vi "模拟发送.vi"() -> ()   [LabVIEW 2013]
panel:
  in  "循环发送帧间隔":dbl
  out "Stop":bool
  in  "内部CAN发送通道":u16(ring) items=["CAN0", "CAN1"]
  in  "加载配置文件":bool
  in  "默认":bool
  in  "开始":bool
  in  "停止":bool
  in  "选项卡控件":enum32{"从板信息", "高压板信息", "故障信息", "自定义信息发送"}(tab)
  in  "温度个数":dbl
  in  "温度":dbl
  in  "电压个数":dbl
  in  "单体电压":dbl
  in  "LIFE":i32
  in  "从板总电压":dbl
  in  "最大电压":dbl
  in  "位置":i32
  in  "最小电压":dbl
  in  "位置":i32
  in  "最大温度":dbl
  in  "位置":i32
  in  "最小温度":dbl
  in  "位置":i32
  in  "从板个数":T1(ring)
  in  "发送单体电压递增1mv":bool
  in  "发送温度递增1度":bool
  in  "板号               单体电压          电压个数":dbl[][](array[numeric])
  in  "板号          温度              温度个数":dbl[][](array[numeric])
  in  "总电压 2":dbl caption="总电压"
  in  "总电流 2":dbl caption="总电流"
  in  "外总压 2":dbl caption="外总压"
  in  "平均电流 2":dbl caption="平均电流"
  in  "充电总安时":dbl
  in  "放电总安时":dbl
  in  "发送?":bool
  in  "电压检测模块故障":enum16{"无", "一级", "二级", "三级"}(ring)
  in  "温度检测模块故障":enum16{"无", "一级", "二级", "三级"}(ring) caption="电压检测模块故障"
  in  "电流检测模块故障":enum16{"无", "一级", "二级", "三级"}(ring) caption="电压检测模块故障"
  in  "绝缘检测模块故障":enum16{"无", "一级", "二级", "三级"}(ring) caption="电压检测模块故障"
  in  "内总压检测模块故障":enum16{"无", "一级", "二级", "三级"}(ring) caption="电压检测模块故障"
  in  "外总压检测模块故障":enum16{"无", "一级", "二级", "三级"}(ring) caption="电压检测模块故障"
  in  "系统外扩时钟模块故障":enum16{"无", "一级", "二级", "三级"}(ring) caption="电压检测模块故障"
  in  "CPU内部EE故障":enum16{"无", "一级", "二级", "三级"}(ring) caption="电压检测模块故障"
  in  "EE存储器故障":enum16{"无", "一级", "二级", "三级"}(ring) caption="电压检测模块故障"
  in  "45db041存储器故障":enum16{"无", "一级", "二级", "三级"}(ring) caption="电压检测模块故障"
  in  "CPU内部FLASH存储器故障":enum16{"无", "一级", "二级", "三级"}(ring) caption="电压检测模块故障"
  in  "CPU故障":enum16{"无", "一级", "二级", "三级"}(ring) caption="电压检测模块故障"
  in  "CAN4通讯模块故障":enum16{"无", "一级", "二级", "三级"}(ring) caption="电压检测模块故障"
  in  "CAN0通讯模块故障":enum16{"无", "一级", "二级", "三级"}(ring) caption="电压检测模块故障"
  in  "CAN1通讯模块故障":enum16{"无", "一级", "二级", "三级"}(ring) caption="电压检测模块故障"
  in  "充电均衡模块故障":enum16{"无", "一级", "二级", "三级"}(ring) caption="电压检测模块故障"
  in  "放电均衡模块故障":enum16{"无", "一级", "二级", "三级"}(ring) caption="电压检测模块故障"
  in  "软件故障":enum16{"无", "一级", "二级", "三级"}(ring) caption="电压检测模块故障"
  in  "DI模块故障":enum16{"无", "一级", "二级", "三级"}(ring) caption="电压检测模块故障"
  in  "DO模块故障":enum16{"无", "一级", "二级", "三级"}(ring) caption="电压检测模块故障"
  in  "全选":bool
  in  "清空":bool
  out "硬件故障":string
  in  "循环发送":bool
  in  "单次发送":bool
  in  "自定信息CAN发送通道":u16(ring) items=["CAN0", "CAN1"]
  in  "自定义数据":string[][](table)
  in  "自定义信息CAN波特率":enum16{"250Kbps", "500Kbps"}(ring)=enum."500Kbps"
  in  "2":bool
  in  "3":bool
  in  "4":bool
  in  "5":bool
  in  "6":bool
  in  "7":bool
  in  "8":bool
  in  "9":bool
  in  "10":bool
  in  "1":bool=TRUE
  out "发送成功":bool
  in  "平均电流":dbl
  in  "外总压":dbl
  in  "总电流":dbl
  # "模拟数据发送"
  # "设置全部从板温度信息"
  # "设置全部从板电压信息"
  # "发送"
  # "双击序号可发送指定帧"
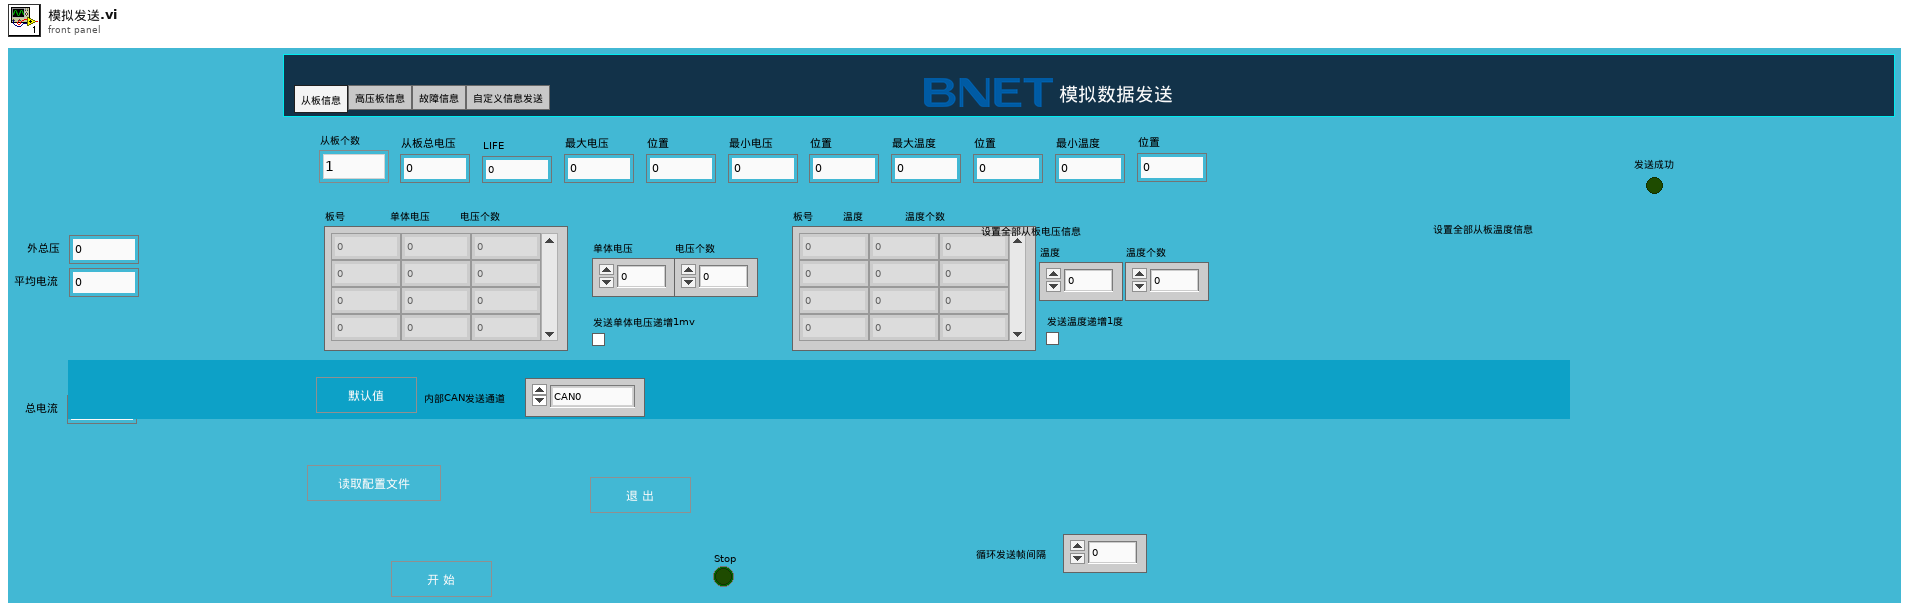
[diagram p1: front panel]
types:
  T1 = enum16{"1", "2", "3", "4", "5", "6", "7", "8", "9", "10", "11", "12", "13", "14", "15", "16", "17", "18", "19", "20", "21", "22", "23", "24", "25", "26", "27", "28", "29", "30"}
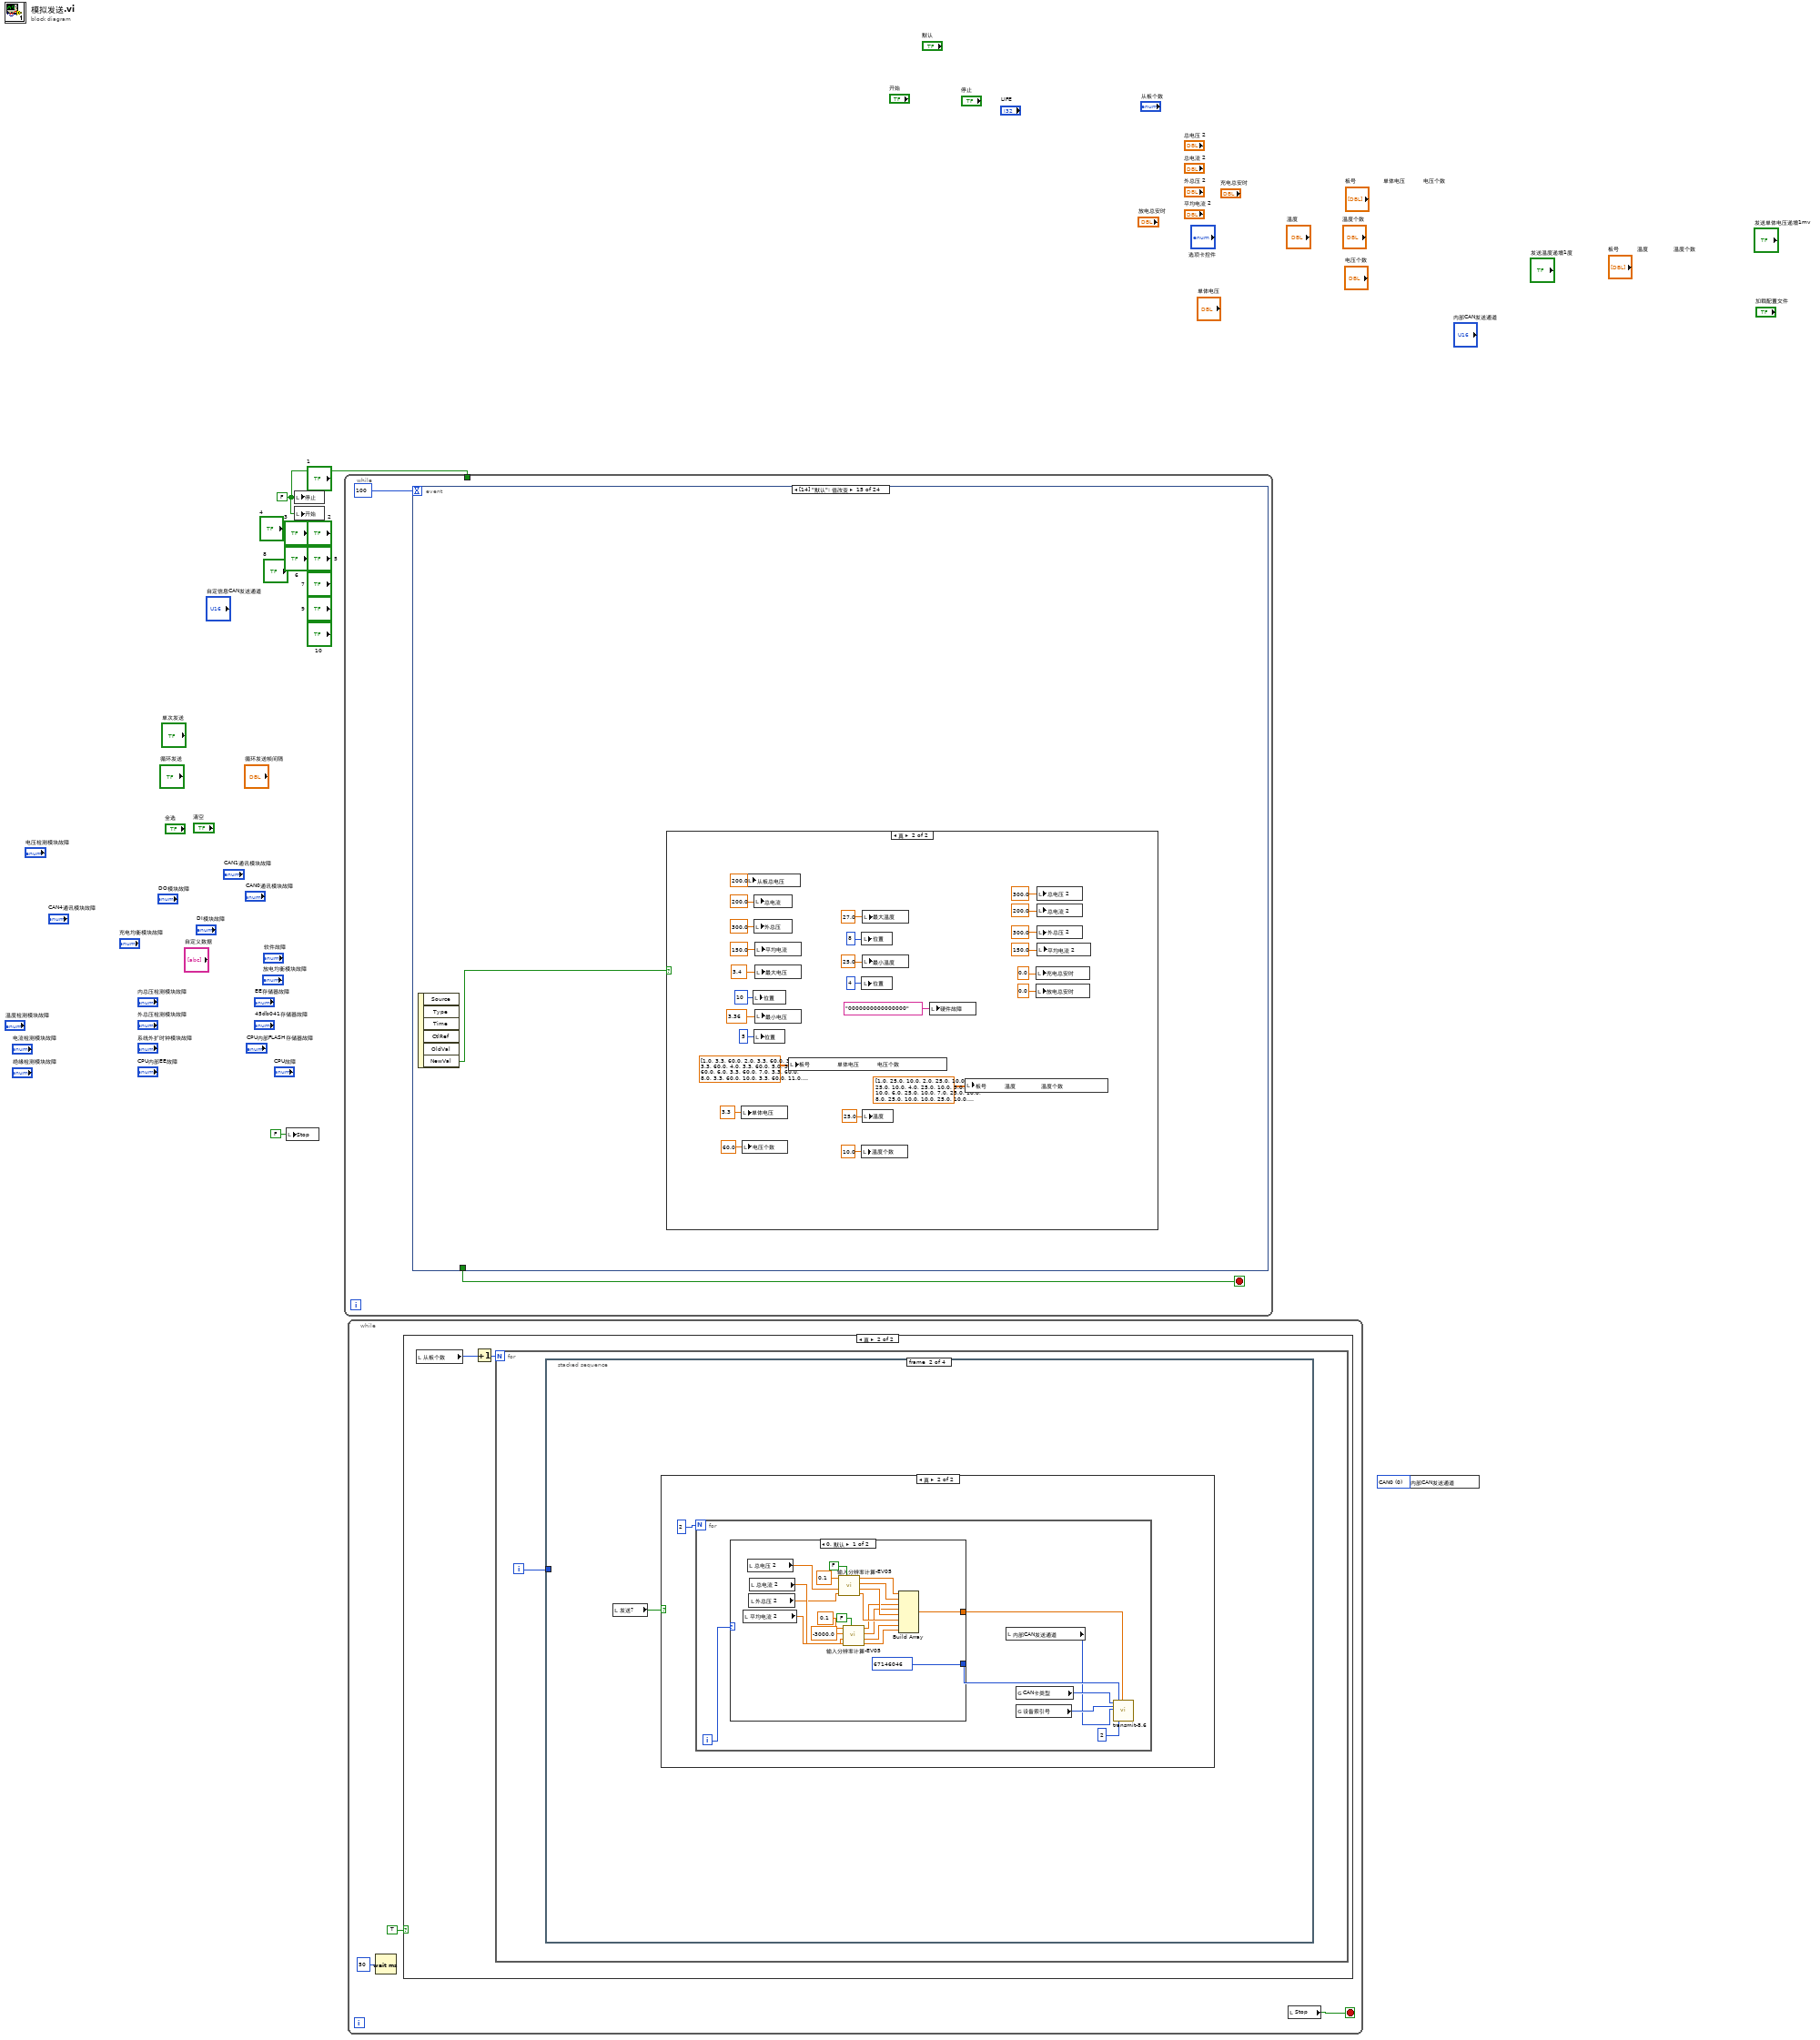
[diagram p0: block diagram]
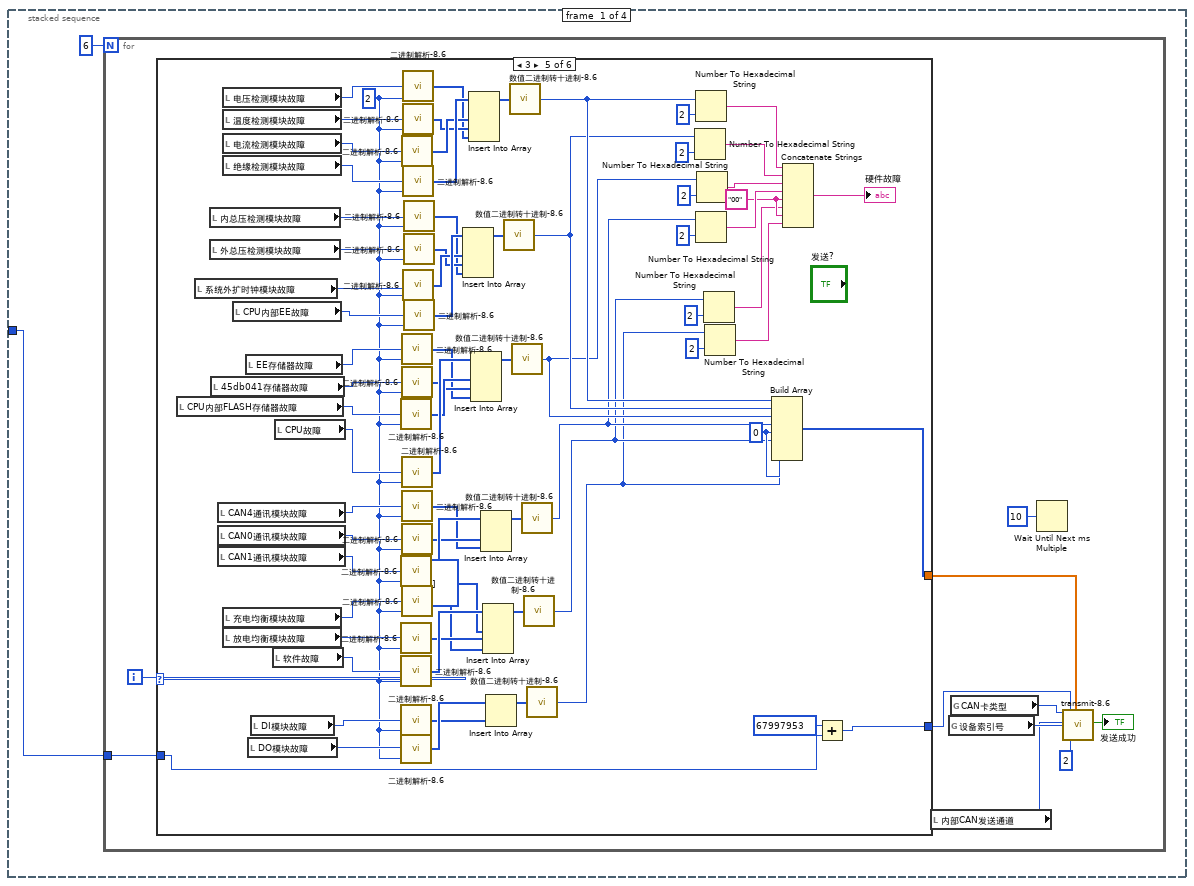
[diagram p3: hidden frame]
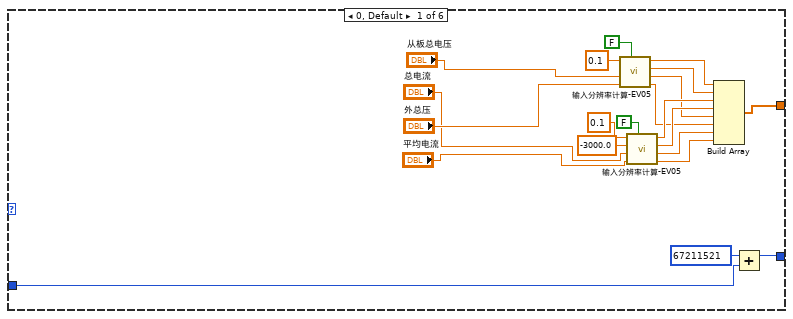
[diagram p4: hidden frame]
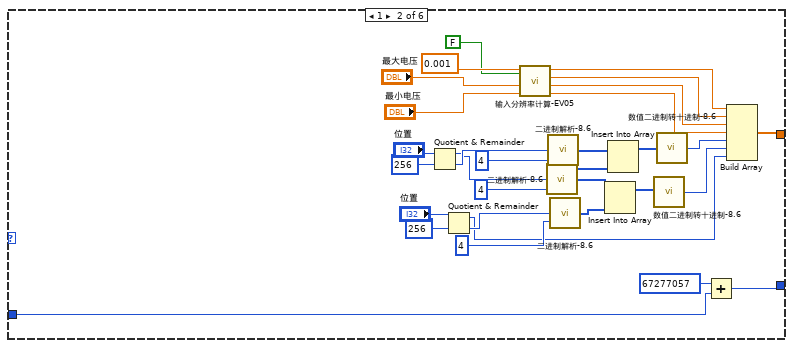
[diagram p5: hidden frame]
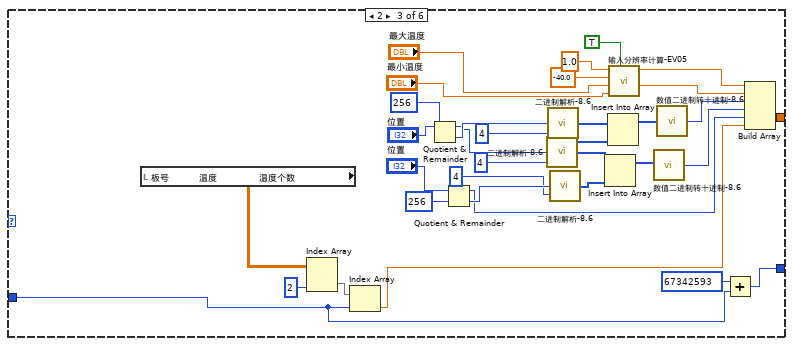
[diagram p6: hidden frame]
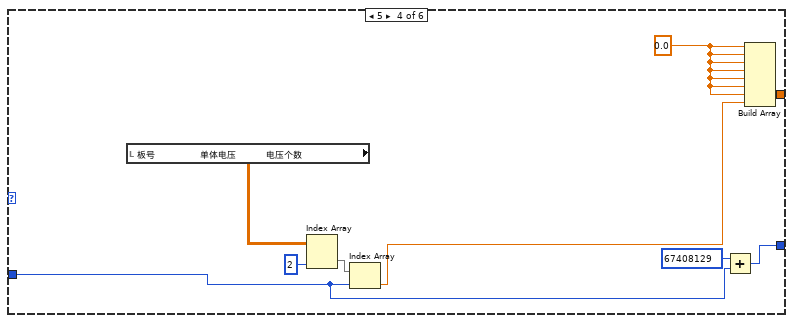
[diagram p7: hidden frame]
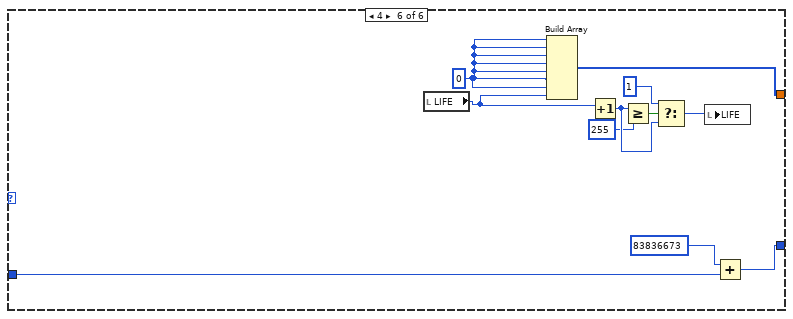
[diagram p8: hidden frame]
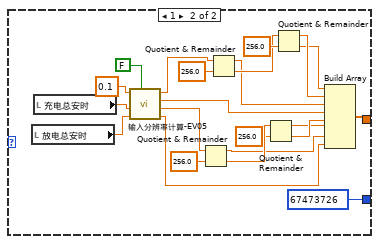
[diagram p10: hidden frame]
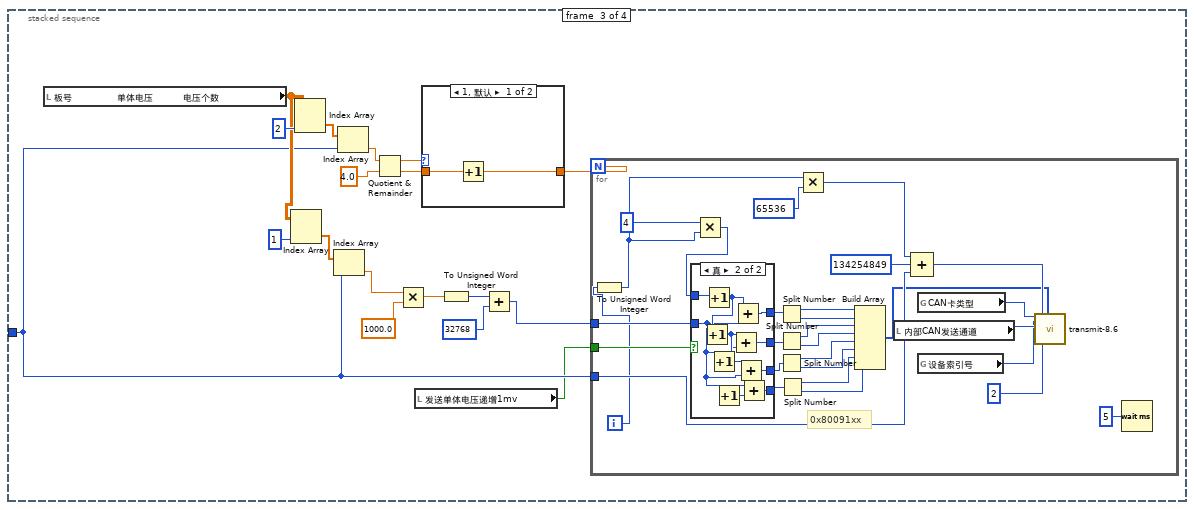
[diagram p11: hidden frame]
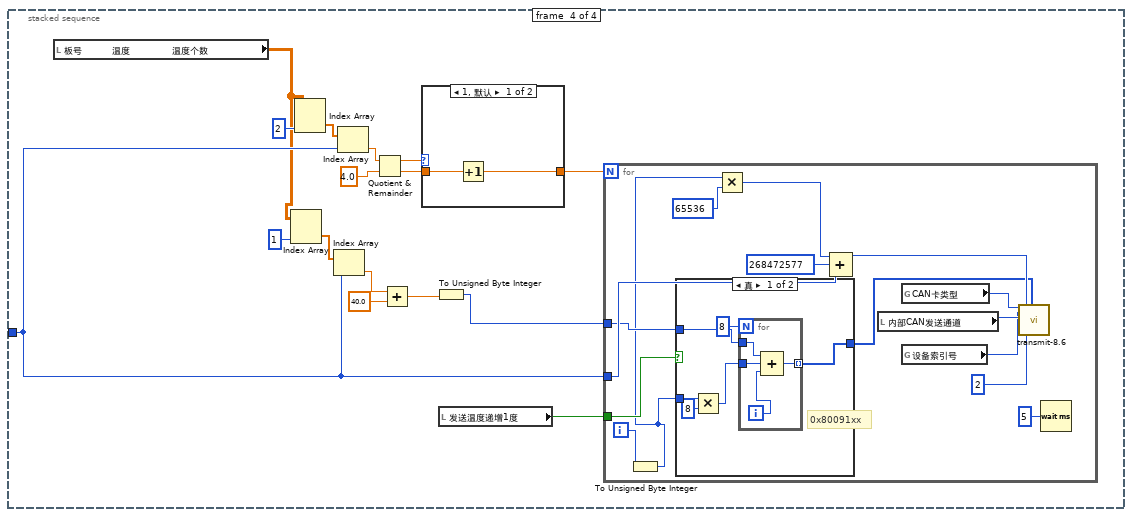
[diagram p14: hidden frame]
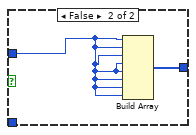
[diagram p16: hidden frame]
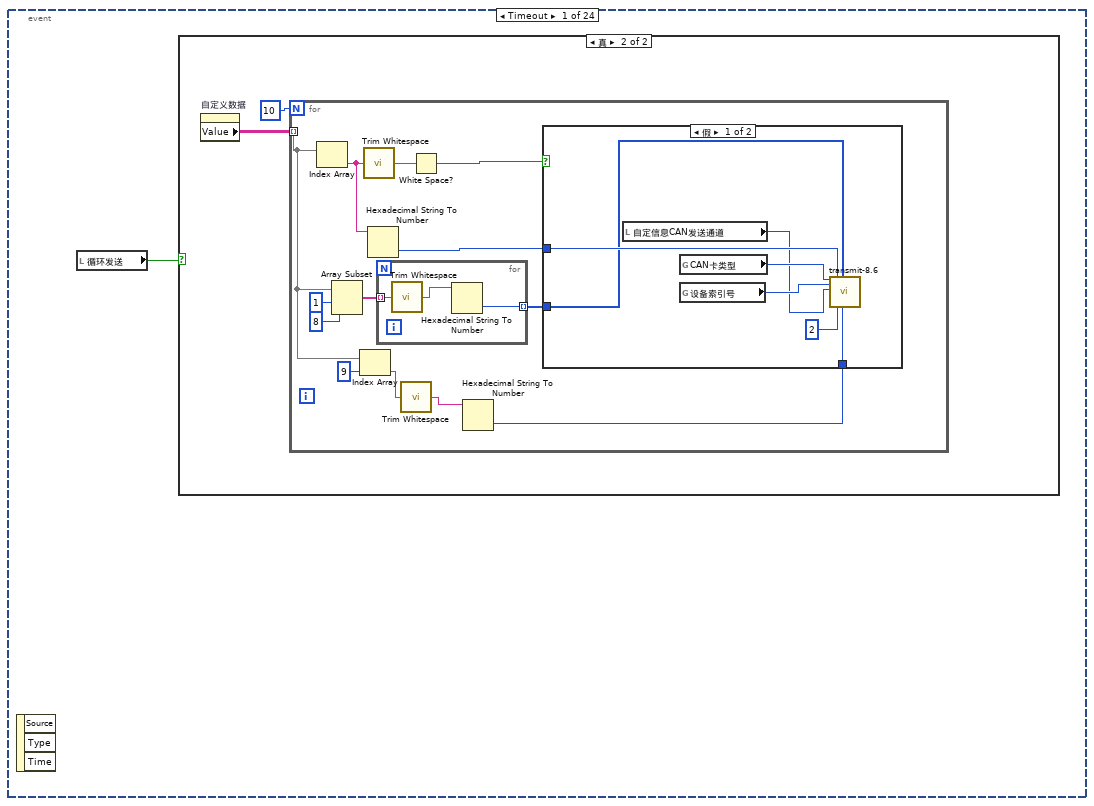
[diagram p17: hidden frame]
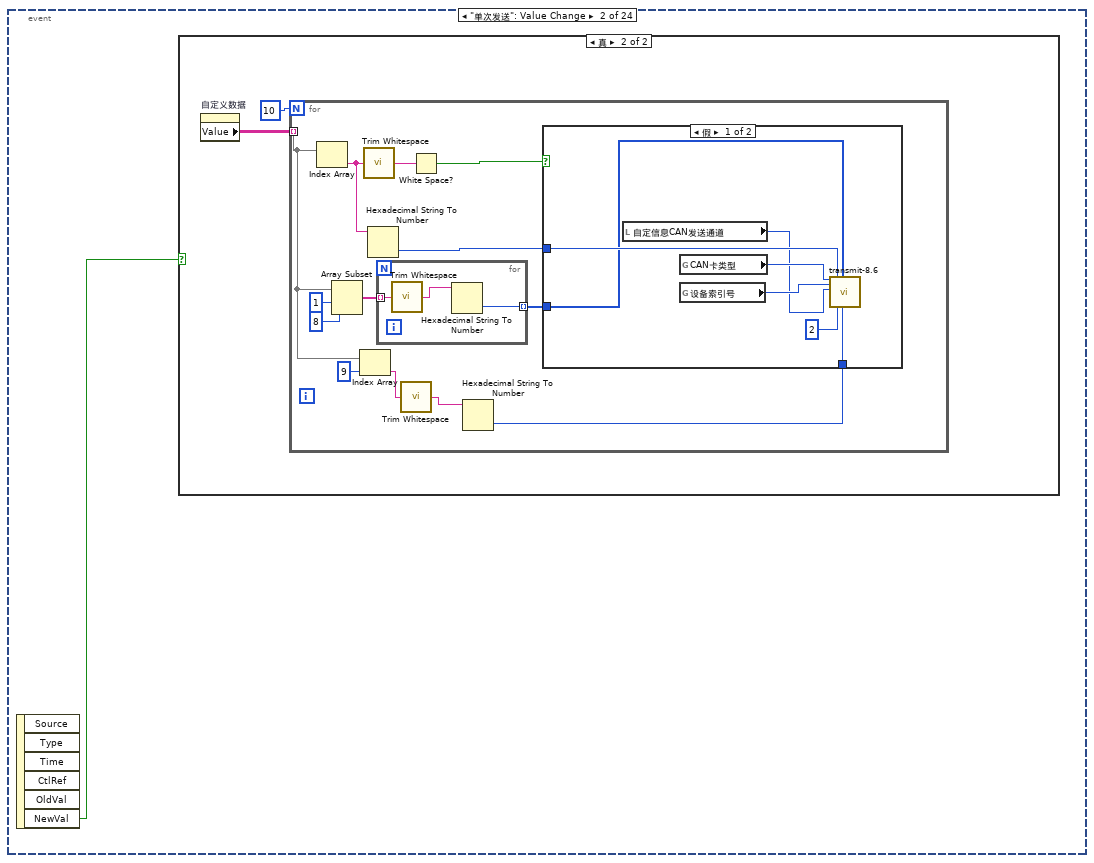
[diagram p20: hidden frame]
diagram:
  w1 = u16 0 items=["CAN0", "CAN1"] ("CAN通道")
  w3 = FALSE ("开始")
  n1 = local write "Stop"(FALSE ("Stop")) -> ()
  n2 = local write "停止"(w3) -> ()
  n3 = local write "开始"(w3) -> ()
  n4 = while {
    tunnel: w3 -> [_]
    stop <- w4 stop-if-true
    n5 = event shown="[14] \"默认\": 值改变" {
      selector: _ -> [_ _ _ _ _ _ _ _ _ _ _ _ _ _ _ _ _ _ _ _ _ _ _ _]
      dyn-events: _ -> [_ _ _ _ _ _ _ _ _ _ _ _ _ _ _ _ _ _ _ _ _ _ _ _]
      timeout: 100 -> [_ _ _ _ _ _ _ _ _ _ _ _ _ _ _ _ _ _ _ _ _ _ _ _]
      tunnel: [_ _ _ _ _ _ _ _ _ _ _ _ _ _ _ _ _ _ _ w396 TRUE ("NewVal") _ _ _] -> w4
      event Timeout {
        n6 = event-data() -> ()  [unwired: 1 in, 3 out]
        n7 = local read "循环发送"() -> (w6:bool)
        n8 = case shown="真" w6 {
          frame False {
          }
          frame True {
            n9 = property on="自定义数据" class="Tbl (严格)"() -> ("Value"=w8:string[][])  [unwired: 2 in, 2 out]
            n10 = for {
              N: 10 -> [_]
              tunnel: w8 -> [w15] mode=indexing
              n11 = Index Array(array=w15) -> (element=w18:string)  [unwired: 1 in]
              n12 = Array Subset(array=w15, index=1 ("索引"), length=8 ("长度")) -> (w10:string[])
              n13 = Index Array(array=w15, index=9 ("索引")) -> (element=w13:string)
              n14 = call <vilib>:"Trim Whitespace.vi"("string"=w18) -> ("trimmed string"=w21:string)  [unwired: 1 in]
              n15 = Hexadecimal String To Number(string=w18) -> (number=w19:u32)  [unwired: 2 in, 1 out]
              n16 = for {
                tunnel: w10 -> [w24] mode=indexing
                tunnel: [w22] -> w9 mode=indexing
                n17 = call <vilib>:"Trim Whitespace.vi"("string"=w24) -> ("trimmed string"=w23:string)  [unwired: 1 in]
                n18 = Hexadecimal String To Number(string=w23) -> (number=w22:u32)  [unwired: 2 in, 1 out]
              }
              n19 = call <vilib>:"Trim Whitespace.vi"("string"=w13) -> ("trimmed string"=w12:string)  [unwired: 1 in]
              n20 = White Space?(1:w21) -> (0:w20:bool)
              n21 = Hexadecimal String To Number(string=w12) -> (number=w11:u32)  [unwired: 2 in, 1 out]
              n22 = case shown="假" w20 {
                tunnel: w19 -> [w28 _]
                tunnel: w11 -> [w27 _]
                tunnel: w9 -> [w26 _]
                frame False {
                  n23 = local read "自定信息CAN发送通道"() -> (w25:u16)
                  n24 = global read "EV05全局变量1.vi" "CAN卡类型"() -> (w31:u32)
                  n25 = global read "EV05全局变量1.vi" "设备索引号"() -> (w30:u16)
                  n26 = call "transmit-8.6.vi"("can卡类型"=w31, "设备索引号"=w30, "CAN端口"=w25, "ID"=w28, "SendType"=u8 2, "Data"=w26, "Eflag"=w27) -> ()  [unwired: 2 in, 11 out]
                }
                frame True {
                }
              }
            }
          }
        }
      }
      event "单次发送": Value Change {
        n27 = event-data() -> ("NewVal"=w32:bool)  [unwired: 1 in, 5 out]
        n28 = case shown="真" w32 {
          frame False {
          }
          frame True {
            n29 = property on="自定义数据" class="Tbl (严格)"() -> ("Value"=w34:string[][])  [unwired: 2 in, 2 out]
            n30 = for {
              N: 10 -> [_]
              tunnel: w34 -> [w41] mode=indexing
              n31 = Index Array(array=w41) -> (element=w44:string)  [unwired: 1 in]
              n32 = Array Subset(array=w41, index=1 ("索引"), length=8 ("长度")) -> (w36:string[])
              n33 = Index Array(array=w41, index=9 ("索引")) -> (element=w39:string)
              n34 = call <vilib>:"Trim Whitespace.vi"("string"=w44) -> ("trimmed string"=w47:string)  [unwired: 1 in]
              n35 = Hexadecimal String To Number(string=w44) -> (number=w45:u32)  [unwired: 2 in, 1 out]
              n36 = for {
                tunnel: w36 -> [w50] mode=indexing
                tunnel: [w48] -> w35 mode=indexing
                n37 = call <vilib>:"Trim Whitespace.vi"("string"=w50) -> ("trimmed string"=w49:string)  [unwired: 1 in]
                n38 = Hexadecimal String To Number(string=w49) -> (number=w48:u32)  [unwired: 2 in, 1 out]
              }
              n39 = call <vilib>:"Trim Whitespace.vi"("string"=w39) -> ("trimmed string"=w38:string)  [unwired: 1 in]
              n40 = White Space?(1:w47) -> (0:w46:bool)
              n41 = Hexadecimal String To Number(string=w38) -> (number=w37:u32)  [unwired: 2 in, 1 out]
              n42 = case shown="假" w46 {
                tunnel: w45 -> [w54 _]
                tunnel: w37 -> [w53 _]
                tunnel: w35 -> [w52 _]
                frame False {
                  n43 = local read "自定信息CAN发送通道"() -> (w51:u16)
                  n44 = global read "EV05全局变量1.vi" "CAN卡类型"() -> (w57:u32)
                  n45 = global read "EV05全局变量1.vi" "设备索引号"() -> (w56:u16)
                  n46 = call "transmit-8.6.vi"("can卡类型"=w57, "设备索引号"=w56, "CAN端口"=w51, "ID"=w54, "SendType"=u8 2, "Data"=w52, "Eflag"=w53) -> ()  [unwired: 2 in, 11 out]
                }
                frame True {
                }
              }
            }
          }
        }
      }
      event "1": Mouse Down {
        n47 = event-data() -> ("CtlRef"=w75:refnum<vi>)  [unwired: 1 in, 7 out]
        n48 = property class="Bool (严格)"(reference=w75) -> ("Label.Text"=w74:string)  [unwired: 1 in, 2 out]
        n49 = property on="自定义数据" class="Tbl (严格)"() -> ("Value"=w59:string[][])  [unwired: 2 in, 2 out]
        n50 = Decimal String To Number(string=w74) -> (number=w73:i32)  [unwired: 2 in, 1 out]
        n51 = Decrement(x=w73) -> (x-1=w72:i32)
        n52 = Index Array(array=w59, index (row)=w72) -> (element=w58:string[])  [unwired: 1 in]
        n53 = Index Array(array=w58) -> (element=w68:string)  [unwired: 1 in]
        n54 = Array Subset(array=w58, index=1 ("索引"), length=8 ("长度")) -> (w61:string[])
        n55 = Index Array(array=w58, index=9 ("索引")) -> (element=w64:string)
        n56 = call <vilib>:"Trim Whitespace.vi"("string"=w68) -> ("trimmed string"=w71:string)  [unwired: 1 in]
        n57 = Hexadecimal String To Number(string=w68) -> (number=w69:u32)  [unwired: 2 in, 1 out]
        n58 = for {
          tunnel: w61 -> [w78] mode=indexing
          tunnel: [w76] -> w60 mode=indexing
          n59 = call <vilib>:"Trim Whitespace.vi"("string"=w78) -> ("trimmed string"=w77:string)  [unwired: 1 in]
          n60 = Hexadecimal String To Number(string=w77) -> (number=w76:u32)  [unwired: 2 in, 1 out]
        }
        n61 = call <vilib>:"Trim Whitespace.vi"("string"=w64) -> ("trimmed string"=w63:string)  [unwired: 1 in]
        n62 = White Space?(1:w71) -> (0:w70:bool)
        n63 = Hexadecimal String To Number(string=w63) -> (number=w62:u32)  [unwired: 2 in, 1 out]
        n64 = case shown="假" w70 {
          tunnel: w69 -> [w82 _]
          tunnel: w62 -> [w81 _]
          tunnel: w60 -> [w80 _]
          frame False {
            n65 = local read "自定信息CAN发送通道"() -> (w79:u16)
            n66 = global read "EV05全局变量1.vi" "CAN卡类型"() -> (w85:u32)
            n67 = global read "EV05全局变量1.vi" "设备索引号"() -> (w84:u16)
            n68 = call "transmit-8.6.vi"("can卡类型"=w85, "设备索引号"=w84, "CAN端口"=w79, "ID"=w82, "SendType"=u8 2, "Data"=w80, "Eflag"=w81) -> ()  [unwired: 2 in, 11 out]
          }
          frame True {
          }
        }
      }
      event "2": Mouse Down {
        n69 = event-data() -> ("CtlRef"=w103:refnum<vi>)  [unwired: 1 in, 7 out]
        n70 = property class="Bool (严格)"(reference=w103) -> ("Label.Text"=w102:string)  [unwired: 1 in, 2 out]
        n71 = property on="自定义数据" class="Tbl (严格)"() -> ("Value"=w87:string[][])  [unwired: 2 in, 2 out]
        n72 = Decimal String To Number(string=w102) -> (number=w101:i32)  [unwired: 2 in, 1 out]
        n73 = Decrement(x=w101) -> (x-1=w100:i32)
        n74 = Index Array(array=w87, index (row)=w100) -> (element=w86:string[])  [unwired: 1 in]
        n75 = Index Array(array=w86) -> (element=w96:string)  [unwired: 1 in]
        n76 = Array Subset(array=w86, index=1 ("索引"), length=8 ("长度")) -> (w89:string[])
        n77 = Index Array(array=w86, index=9 ("索引")) -> (element=w92:string)
        n78 = call <vilib>:"Trim Whitespace.vi"("string"=w96) -> ("trimmed string"=w99:string)  [unwired: 1 in]
        n79 = Hexadecimal String To Number(string=w96) -> (number=w97:u32)  [unwired: 2 in, 1 out]
        n80 = for {
          tunnel: w89 -> [w106] mode=indexing
          tunnel: [w104] -> w88 mode=indexing
          n81 = call <vilib>:"Trim Whitespace.vi"("string"=w106) -> ("trimmed string"=w105:string)  [unwired: 1 in]
          n82 = Hexadecimal String To Number(string=w105) -> (number=w104:u32)  [unwired: 2 in, 1 out]
        }
        n83 = call <vilib>:"Trim Whitespace.vi"("string"=w92) -> ("trimmed string"=w91:string)  [unwired: 1 in]
        n84 = White Space?(1:w99) -> (0:w98:bool)
        n85 = Hexadecimal String To Number(string=w91) -> (number=w90:u32)  [unwired: 2 in, 1 out]
        n86 = case shown="假" w98 {
          tunnel: w97 -> [w110 _]
          tunnel: w90 -> [w109 _]
          tunnel: w88 -> [w108 _]
          frame False {
            n87 = local read "自定信息CAN发送通道"() -> (w107:u16)
            n88 = global read "EV05全局变量1.vi" "CAN卡类型"() -> (w113:u32)
            n89 = global read "EV05全局变量1.vi" "设备索引号"() -> (w112:u16)
            n90 = call "transmit-8.6.vi"("can卡类型"=w113, "设备索引号"=w112, "CAN端口"=w107, "ID"=w110, "SendType"=u8 2, "Data"=w108, "Eflag"=w109) -> ()  [unwired: 2 in, 11 out]
          }
          frame True {
          }
        }
      }
      event "3": Mouse Down {
        n91 = event-data() -> ("CtlRef"=w131:refnum<vi>)  [unwired: 1 in, 7 out]
        n92 = property class="Bool (严格)"(reference=w131) -> ("Label.Text"=w130:string)  [unwired: 1 in, 2 out]
        n93 = property on="自定义数据" class="Tbl (严格)"() -> ("Value"=w115:string[][])  [unwired: 2 in, 2 out]
        n94 = Decimal String To Number(string=w130) -> (number=w129:i32)  [unwired: 2 in, 1 out]
        n95 = Decrement(x=w129) -> (x-1=w128:i32)
        n96 = Index Array(array=w115, index (row)=w128) -> (element=w114:string[])  [unwired: 1 in]
        n97 = Index Array(array=w114) -> (element=w124:string)  [unwired: 1 in]
        n98 = Array Subset(array=w114, index=1 ("索引"), length=8 ("长度")) -> (w117:string[])
        n99 = Index Array(array=w114, index=9 ("索引")) -> (element=w120:string)
        n100 = call <vilib>:"Trim Whitespace.vi"("string"=w124) -> ("trimmed string"=w127:string)  [unwired: 1 in]
        n101 = Hexadecimal String To Number(string=w124) -> (number=w125:u32)  [unwired: 2 in, 1 out]
        n102 = for {
          tunnel: w117 -> [w134] mode=indexing
          tunnel: [w132] -> w116 mode=indexing
          n103 = call <vilib>:"Trim Whitespace.vi"("string"=w134) -> ("trimmed string"=w133:string)  [unwired: 1 in]
          n104 = Hexadecimal String To Number(string=w133) -> (number=w132:u32)  [unwired: 2 in, 1 out]
        }
        n105 = call <vilib>:"Trim Whitespace.vi"("string"=w120) -> ("trimmed string"=w119:string)  [unwired: 1 in]
        n106 = White Space?(1:w127) -> (0:w126:bool)
        n107 = Hexadecimal String To Number(string=w119) -> (number=w118:u32)  [unwired: 2 in, 1 out]
        n108 = case shown="假" w126 {
          tunnel: w125 -> [w138 _]
          tunnel: w118 -> [w137 _]
          tunnel: w116 -> [w136 _]
          frame False {
            n109 = local read "自定信息CAN发送通道"() -> (w135:u16)
            n110 = global read "EV05全局变量1.vi" "CAN卡类型"() -> (w141:u32)
            n111 = global read "EV05全局变量1.vi" "设备索引号"() -> (w140:u16)
            n112 = call "transmit-8.6.vi"("can卡类型"=w141, "设备索引号"=w140, "CAN端口"=w135, "ID"=w138, "SendType"=u8 2, "Data"=w136, "Eflag"=w137) -> ()  [unwired: 2 in, 11 out]
          }
          frame True {
          }
        }
      }
      event "4": Mouse Down {
        n113 = event-data() -> ("CtlRef"=w159:refnum<vi>)  [unwired: 1 in, 7 out]
        n114 = property class="Bool (严格)"(reference=w159) -> ("Label.Text"=w158:string)  [unwired: 1 in, 2 out]
        n115 = property on="自定义数据" class="Tbl (严格)"() -> ("Value"=w143:string[][])  [unwired: 2 in, 2 out]
        n116 = Decimal String To Number(string=w158) -> (number=w157:i32)  [unwired: 2 in, 1 out]
        n117 = Decrement(x=w157) -> (x-1=w156:i32)
        n118 = Index Array(array=w143, index (row)=w156) -> (element=w142:string[])  [unwired: 1 in]
        n119 = Index Array(array=w142) -> (element=w152:string)  [unwired: 1 in]
        n120 = Array Subset(array=w142, index=1 ("索引"), length=8 ("长度")) -> (w145:string[])
        n121 = Index Array(array=w142, index=9 ("索引")) -> (element=w148:string)
        n122 = call <vilib>:"Trim Whitespace.vi"("string"=w152) -> ("trimmed string"=w155:string)  [unwired: 1 in]
        n123 = Hexadecimal String To Number(string=w152) -> (number=w153:u32)  [unwired: 2 in, 1 out]
        n124 = for {
          tunnel: w145 -> [w162] mode=indexing
          tunnel: [w160] -> w144 mode=indexing
          n125 = call <vilib>:"Trim Whitespace.vi"("string"=w162) -> ("trimmed string"=w161:string)  [unwired: 1 in]
          n126 = Hexadecimal String To Number(string=w161) -> (number=w160:u32)  [unwired: 2 in, 1 out]
        }
        n127 = call <vilib>:"Trim Whitespace.vi"("string"=w148) -> ("trimmed string"=w147:string)  [unwired: 1 in]
        n128 = White Space?(1:w155) -> (0:w154:bool)
        n129 = Hexadecimal String To Number(string=w147) -> (number=w146:u32)  [unwired: 2 in, 1 out]
        n130 = case shown="假" w154 {
          tunnel: w153 -> [w166 _]
          tunnel: w146 -> [w165 _]
          tunnel: w144 -> [w164 _]
          frame False {
            n131 = local read "自定信息CAN发送通道"() -> (w163:u16)
            n132 = global read "EV05全局变量1.vi" "CAN卡类型"() -> (w169:u32)
            n133 = global read "EV05全局变量1.vi" "设备索引号"() -> (w168:u16)
            n134 = call "transmit-8.6.vi"("can卡类型"=w169, "设备索引号"=w168, "CAN端口"=w163, "ID"=w166, "SendType"=u8 2, "Data"=w164, "Eflag"=w165) -> ()  [unwired: 2 in, 11 out]
          }
          frame True {
          }
        }
      }
      event "5": Value Change {
        n135 = event-data() -> ("CtlRef"=w187:refnum<vi>)  [unwired: 1 in, 3 out]
        n136 = property class="Bool (严格)"(reference=w187) -> ("Label.Text"=w186:string)  [unwired: 1 in, 2 out]
        n137 = property on="自定义数据" class="Tbl (严格)"() -> ("Value"=w171:string[][])  [unwired: 2 in, 2 out]
        n138 = Decimal String To Number(string=w186) -> (number=w185:i32)  [unwired: 2 in, 1 out]
        n139 = Decrement(x=w185) -> (x-1=w184:i32)
        n140 = Index Array(array=w171, index (row)=w184) -> (element=w170:string[])  [unwired: 1 in]
        n141 = Index Array(array=w170) -> (element=w180:string)  [unwired: 1 in]
        n142 = Array Subset(array=w170, index=1 ("索引"), length=8 ("长度")) -> (w173:string[])
        n143 = Index Array(array=w170, index=9 ("索引")) -> (element=w176:string)
        n144 = call <vilib>:"Trim Whitespace.vi"("string"=w180) -> ("trimmed string"=w183:string)  [unwired: 1 in]
        n145 = Hexadecimal String To Number(string=w180) -> (number=w181:u32)  [unwired: 2 in, 1 out]
        n146 = for {
          tunnel: w173 -> [w190] mode=indexing
          tunnel: [w188] -> w172 mode=indexing
          n147 = call <vilib>:"Trim Whitespace.vi"("string"=w190) -> ("trimmed string"=w189:string)  [unwired: 1 in]
          n148 = Hexadecimal String To Number(string=w189) -> (number=w188:u32)  [unwired: 2 in, 1 out]
        }
        n149 = call <vilib>:"Trim Whitespace.vi"("string"=w176) -> ("trimmed string"=w175:string)  [unwired: 1 in]
        n150 = White Space?(1:w183) -> (0:w182:bool)
        n151 = Hexadecimal String To Number(string=w175) -> (number=w174:u32)  [unwired: 2 in, 1 out]
        n152 = case shown="假" w182 {
          tunnel: w181 -> [w194 _]
          tunnel: w174 -> [w193 _]
          tunnel: w172 -> [w192 _]
          frame False {
            n153 = local read "自定信息CAN发送通道"() -> (w191:u16)
            n154 = global read "EV05全局变量1.vi" "CAN卡类型"() -> (w197:u32)
            n155 = global read "EV05全局变量1.vi" "设备索引号"() -> (w196:u16)
            n156 = call "transmit-8.6.vi"("can卡类型"=w197, "设备索引号"=w196, "CAN端口"=w191, "ID"=w194, "SendType"=u8 2, "Data"=w192, "Eflag"=w193) -> ()  [unwired: 2 in, 11 out]
          }
          frame True {
          }
        }
      }
      event "6": Value Change {
        n157 = event-data() -> ("CtlRef"=w215:refnum<vi>)  [unwired: 1 in, 3 out]
        n158 = property class="Bool (严格)"(reference=w215) -> ("Label.Text"=w214:string)  [unwired: 1 in, 2 out]
        n159 = property on="自定义数据" class="Tbl (严格)"() -> ("Value"=w199:string[][])  [unwired: 2 in, 2 out]
        n160 = Decimal String To Number(string=w214) -> (number=w213:i32)  [unwired: 2 in, 1 out]
        n161 = Decrement(x=w213) -> (x-1=w212:i32)
        n162 = Index Array(array=w199, index (row)=w212) -> (element=w198:string[])  [unwired: 1 in]
        n163 = Index Array(array=w198) -> (element=w208:string)  [unwired: 1 in]
        n164 = Array Subset(array=w198, index=1 ("索引"), length=8 ("长度")) -> (w201:string[])
        n165 = Index Array(array=w198, index=9 ("索引")) -> (element=w204:string)
        n166 = call <vilib>:"Trim Whitespace.vi"("string"=w208) -> ("trimmed string"=w211:string)  [unwired: 1 in]
        n167 = Hexadecimal String To Number(string=w208) -> (number=w209:u32)  [unwired: 2 in, 1 out]
        n168 = for {
          tunnel: w201 -> [w218] mode=indexing
          tunnel: [w216] -> w200 mode=indexing
          n169 = call <vilib>:"Trim Whitespace.vi"("string"=w218) -> ("trimmed string"=w217:string)  [unwired: 1 in]
          n170 = Hexadecimal String To Number(string=w217) -> (number=w216:u32)  [unwired: 2 in, 1 out]
        }
        n171 = call <vilib>:"Trim Whitespace.vi"("string"=w204) -> ("trimmed string"=w203:string)  [unwired: 1 in]
        n172 = White Space?(1:w211) -> (0:w210:bool)
        n173 = Hexadecimal String To Number(string=w203) -> (number=w202:u32)  [unwired: 2 in, 1 out]
        n174 = case shown="假" w210 {
          tunnel: w209 -> [w222 _]
          tunnel: w202 -> [w221 _]
          tunnel: w200 -> [w220 _]
          frame False {
            n175 = local read "自定信息CAN发送通道"() -> (w219:u16)
            n176 = global read "EV05全局变量1.vi" "CAN卡类型"() -> (w225:u32)
            n177 = global read "EV05全局变量1.vi" "设备索引号"() -> (w224:u16)
            n178 = call "transmit-8.6.vi"("can卡类型"=w225, "设备索引号"=w224, "CAN端口"=w219, "ID"=w222, "SendType"=u8 2, "Data"=w220, "Eflag"=w221) -> ()  [unwired: 2 in, 11 out]
          }
          frame True {
          }
        }
      }
      event "7": Value Change {
        n179 = event-data() -> ("CtlRef"=w243:refnum<vi>)  [unwired: 1 in, 3 out]
        n180 = property class="Bool (严格)"(reference=w243) -> ("Label.Text"=w242:string)  [unwired: 1 in, 2 out]
        n181 = property on="自定义数据" class="Tbl (严格)"() -> ("Value"=w227:string[][])  [unwired: 2 in, 2 out]
        n182 = Decimal String To Number(string=w242) -> (number=w241:i32)  [unwired: 2 in, 1 out]
        n183 = Decrement(x=w241) -> (x-1=w240:i32)
        n184 = Index Array(array=w227, index (row)=w240) -> (element=w226:string[])  [unwired: 1 in]
        n185 = Index Array(array=w226) -> (element=w236:string)  [unwired: 1 in]
        n186 = Array Subset(array=w226, index=1 ("索引"), length=8 ("长度")) -> (w229:string[])
        n187 = Index Array(array=w226, index=9 ("索引")) -> (element=w232:string)
        n188 = call <vilib>:"Trim Whitespace.vi"("string"=w236) -> ("trimmed string"=w239:string)  [unwired: 1 in]
        n189 = Hexadecimal String To Number(string=w236) -> (number=w237:u32)  [unwired: 2 in, 1 out]
        n190 = for {
          tunnel: w229 -> [w246] mode=indexing
          tunnel: [w244] -> w228 mode=indexing
          n191 = call <vilib>:"Trim Whitespace.vi"("string"=w246) -> ("trimmed string"=w245:string)  [unwired: 1 in]
          n192 = Hexadecimal String To Number(string=w245) -> (number=w244:u32)  [unwired: 2 in, 1 out]
        }
        n193 = call <vilib>:"Trim Whitespace.vi"("string"=w232) -> ("trimmed string"=w231:string)  [unwired: 1 in]
        n194 = White Space?(1:w239) -> (0:w238:bool)
        n195 = Hexadecimal String To Number(string=w231) -> (number=w230:u32)  [unwired: 2 in, 1 out]
        n196 = case shown="假" w238 {
          tunnel: w237 -> [w250 _]
          tunnel: w230 -> [w249 _]
          tunnel: w228 -> [w248 _]
          frame False {
            n197 = local read "自定信息CAN发送通道"() -> (w247:u16)
            n198 = global read "EV05全局变量1.vi" "CAN卡类型"() -> (w253:u32)
            n199 = global read "EV05全局变量1.vi" "设备索引号"() -> (w252:u16)
            n200 = call "transmit-8.6.vi"("can卡类型"=w253, "设备索引号"=w252, "CAN端口"=w247, "ID"=w250, "SendType"=u8 2, "Data"=w248, "Eflag"=w249) -> ()  [unwired: 2 in, 11 out]
          }
          frame True {
          }
        }
      }
      event "8": Value Change {
        n201 = event-data() -> ("CtlRef"=w271:refnum<vi>)  [unwired: 1 in, 3 out]
        n202 = property class="Bool (严格)"(reference=w271) -> ("Label.Text"=w270:string)  [unwired: 1 in, 2 out]
        n203 = property on="自定义数据" class="Tbl (严格)"() -> ("Value"=w255:string[][])  [unwired: 2 in, 2 out]
        n204 = Decimal String To Number(string=w270) -> (number=w269:i32)  [unwired: 2 in, 1 out]
        n205 = Decrement(x=w269) -> (x-1=w268:i32)
        n206 = Index Array(array=w255, index (row)=w268) -> (element=w254:string[])  [unwired: 1 in]
        n207 = Index Array(array=w254) -> (element=w264:string)  [unwired: 1 in]
        n208 = Array Subset(array=w254, index=1 ("索引"), length=8 ("长度")) -> (w257:string[])
        n209 = Index Array(array=w254, index=9 ("索引")) -> (element=w260:string)
        n210 = call <vilib>:"Trim Whitespace.vi"("string"=w264) -> ("trimmed string"=w267:string)  [unwired: 1 in]
        n211 = Hexadecimal String To Number(string=w264) -> (number=w265:u32)  [unwired: 2 in, 1 out]
        n212 = for {
          tunnel: w257 -> [w274] mode=indexing
          tunnel: [w272] -> w256 mode=indexing
          n213 = call <vilib>:"Trim Whitespace.vi"("string"=w274) -> ("trimmed string"=w273:string)  [unwired: 1 in]
          n214 = Hexadecimal String To Number(string=w273) -> (number=w272:u32)  [unwired: 2 in, 1 out]
        }
        n215 = call <vilib>:"Trim Whitespace.vi"("string"=w260) -> ("trimmed string"=w259:string)  [unwired: 1 in]
        n216 = White Space?(1:w267) -> (0:w266:bool)
        n217 = Hexadecimal String To Number(string=w259) -> (number=w258:u32)  [unwired: 2 in, 1 out]
        n218 = case shown="假" w266 {
          tunnel: w265 -> [w278 _]
          tunnel: w258 -> [w277 _]
          tunnel: w256 -> [w276 _]
          frame False {
            n219 = local read "自定信息CAN发送通道"() -> (w275:u16)
            n220 = global read "EV05全局变量1.vi" "CAN卡类型"() -> (w281:u32)
            n221 = global read "EV05全局变量1.vi" "设备索引号"() -> (w280:u16)
            n222 = call "transmit-8.6.vi"("can卡类型"=w281, "设备索引号"=w280, "CAN端口"=w275, "ID"=w278, "SendType"=u8 2, "Data"=w276, "Eflag"=w277) -> ()  [unwired: 2 in, 11 out]
          }
          frame True {
          }
        }
      }
      event "9": Value Change {
        n223 = event-data() -> ("CtlRef"=w299:refnum<vi>)  [unwired: 1 in, 3 out]
        n224 = property class="Bool (严格)"(reference=w299) -> ("Label.Text"=w298:string)  [unwired: 1 in, 2 out]
        n225 = property on="自定义数据" class="Tbl (严格)"() -> ("Value"=w283:string[][])  [unwired: 2 in, 2 out]
        n226 = Decimal String To Number(string=w298) -> (number=w297:i32)  [unwired: 2 in, 1 out]
        n227 = Decrement(x=w297) -> (x-1=w296:i32)
        n228 = Index Array(array=w283, index (row)=w296) -> (element=w282:string[])  [unwired: 1 in]
        n229 = Index Array(array=w282) -> (element=w292:string)  [unwired: 1 in]
        n230 = Array Subset(array=w282, index=1 ("索引"), length=8 ("长度")) -> (w285:string[])
        n231 = Index Array(array=w282, index=9 ("索引")) -> (element=w288:string)
        n232 = call <vilib>:"Trim Whitespace.vi"("string"=w292) -> ("trimmed string"=w295:string)  [unwired: 1 in]
        n233 = Hexadecimal String To Number(string=w292) -> (number=w293:u32)  [unwired: 2 in, 1 out]
        n234 = for {
          tunnel: w285 -> [w302] mode=indexing
          tunnel: [w300] -> w284 mode=indexing
          n235 = call <vilib>:"Trim Whitespace.vi"("string"=w302) -> ("trimmed string"=w301:string)  [unwired: 1 in]
          n236 = Hexadecimal String To Number(string=w301) -> (number=w300:u32)  [unwired: 2 in, 1 out]
        }
        n237 = call <vilib>:"Trim Whitespace.vi"("string"=w288) -> ("trimmed string"=w287:string)  [unwired: 1 in]
        n238 = White Space?(1:w295) -> (0:w294:bool)
        n239 = Hexadecimal String To Number(string=w287) -> (number=w286:u32)  [unwired: 2 in, 1 out]
        n240 = case shown="假" w294 {
          tunnel: w293 -> [w306 _]
          tunnel: w286 -> [w305 _]
          tunnel: w284 -> [w304 _]
          frame False {
            n241 = local read "自定信息CAN发送通道"() -> (w303:u16)
            n242 = global read "EV05全局变量1.vi" "CAN卡类型"() -> (w309:u32)
            n243 = global read "EV05全局变量1.vi" "设备索引号"() -> (w308:u16)
            n244 = call "transmit-8.6.vi"("can卡类型"=w309, "设备索引号"=w308, "CAN端口"=w303, "ID"=w306, "SendType"=u8 2, "Data"=w304, "Eflag"=w305) -> ()  [unwired: 2 in, 11 out]
          }
          frame True {
          }
        }
      }
      event "10": Value Change {
        n245 = event-data() -> ("CtlRef"=w327:refnum<vi>)  [unwired: 1 in, 3 out]
        n246 = property class="Bool (严格)"(reference=w327) -> ("Label.Text"=w326:string)  [unwired: 1 in, 2 out]
        n247 = property on="自定义数据" class="Tbl (严格)"() -> ("Value"=w311:string[][])  [unwired: 2 in, 2 out]
        n248 = Decimal String To Number(string=w326) -> (number=w325:i32)  [unwired: 2 in, 1 out]
        n249 = Decrement(x=w325) -> (x-1=w324:i32)
        n250 = Index Array(array=w311, index (row)=w324) -> (element=w310:string[])  [unwired: 1 in]
        n251 = Index Array(array=w310) -> (element=w320:string)  [unwired: 1 in]
        n252 = Array Subset(array=w310, index=1 ("索引"), length=8 ("长度")) -> (w313:string[])
        n253 = Index Array(array=w310, index=9 ("索引")) -> (element=w316:string)
        n254 = call <vilib>:"Trim Whitespace.vi"("string"=w320) -> ("trimmed string"=w323:string)  [unwired: 1 in]
        n255 = Hexadecimal String To Number(string=w320) -> (number=w321:u32)  [unwired: 2 in, 1 out]
        n256 = for {
          tunnel: w313 -> [w330] mode=indexing
          tunnel: [w328] -> w312 mode=indexing
          n257 = call <vilib>:"Trim Whitespace.vi"("string"=w330) -> ("trimmed string"=w329:string)  [unwired: 1 in]
          n258 = Hexadecimal String To Number(string=w329) -> (number=w328:u32)  [unwired: 2 in, 1 out]
        }
        n259 = call <vilib>:"Trim Whitespace.vi"("string"=w316) -> ("trimmed string"=w315:string)  [unwired: 1 in]
        n260 = White Space?(1:w323) -> (0:w322:bool)
        n261 = Hexadecimal String To Number(string=w315) -> (number=w314:u32)  [unwired: 2 in, 1 out]
        n262 = case shown="假" w322 {
          tunnel: w321 -> [w334 _]
          tunnel: w314 -> [w333 _]
          tunnel: w312 -> [w332 _]
          frame False {
            n263 = local read "自定信息CAN发送通道"() -> (w331:u16)
            n264 = global read "EV05全局变量1.vi" "CAN卡类型"() -> (w337:u32)
            n265 = global read "EV05全局变量1.vi" "设备索引号"() -> (w336:u16)
            n266 = call "transmit-8.6.vi"("can卡类型"=w337, "设备索引号"=w336, "CAN端口"=w331, "ID"=w334, "SendType"=u8 2, "Data"=w332, "Eflag"=w333) -> ()  [unwired: 2 in, 11 out]
          }
          frame True {
          }
        }
      }
      event "全选": Value Change {
        n267 = event-data() -> ("NewVal"=w338:bool)  [unwired: 1 in, 5 out]
        n268 = case shown="真" w338 {
          frame False {
          }
          frame True {
            w339 = 1
            n269 = local write "CPU内部FLASH存储器故障"(w339) -> ()
            n270 = local write "CPU故障"(w339) -> ()
            n271 = local write "CPU内部EE故障"(w339) -> ()
            n272 = local write "EE存储器故障"(w339) -> ()
            n273 = local write "45db041存储器故障"(w339) -> ()
            n274 = local write "电压检测模块故障"(w339) -> ()
            n275 = local write "电流检测模块故障"(w339) -> ()
            n276 = local write "绝缘检测模块故障"(w339) -> ()
            n277 = local write "CAN4通讯模块故障"(w339) -> ()
            n278 = local write "DO模块故障"(w339) -> ()
            n279 = local write "温度检测模块故障"(w339) -> ()
            n280 = local write "内总压检测模块故障"(w339) -> ()
            n281 = local write "外总压检测模块故障"(w339) -> ()
            n282 = local write "CAN0通讯模块故障"(w339) -> ()
            n283 = local write "CAN1通讯模块故障"(w339) -> ()
            n284 = local write "软件故障"(w339) -> ()
            n285 = local write "系统外扩时钟模块故障"(w339) -> ()
            n286 = local write "充电均衡模块故障"(w339) -> ()
            n287 = local write "放电均衡模块故障"(w339) -> ()
            n288 = local write "DI模块故障"(w339) -> ()
          }
        }
      }
      event "清空": Value Change {
        n289 = event-data() -> ("NewVal"=w340:bool)  [unwired: 1 in, 5 out]
        n290 = case shown="真" w340 {
          frame False {
          }
          frame True {
            w341 = 0
            n291 = local write "CPU故障"(w341) -> ()
            n292 = local write "CPU内部EE故障"(w341) -> ()
            n293 = local write "EE存储器故障"(w341) -> ()
            n294 = local write "45db041存储器故障"(w341) -> ()
            n295 = local write "电压检测模块故障"(w341) -> ()
            n296 = local write "电流检测模块故障"(w341) -> ()
            n297 = local write "绝缘检测模块故障"(w341) -> ()
            n298 = local write "CAN4通讯模块故障"(w341) -> ()
            n299 = local write "DO模块故障"(w341) -> ()
            n300 = local write "温度检测模块故障"(w341) -> ()
            n301 = local write "内总压检测模块故障"(w341) -> ()
            n302 = local write "外总压检测模块故障"(w341) -> ()
            n303 = local write "CAN0通讯模块故障"(w341) -> ()
            n304 = local write "CAN1通讯模块故障"(w341) -> ()
            n305 = local write "软件故障"(w341) -> ()
            n306 = local write "系统外扩时钟模块故障"(w341) -> ()
            n307 = local write "充电均衡模块故障"(w341) -> ()
            n308 = local write "放电均衡模块故障"(w341) -> ()
            n309 = local write "DI模块故障"(w341) -> ()
            n310 = local write "CPU内部FLASH存储器故障"(w341) -> ()
          }
        }
      }
      event "默认": Value Change {
        n311 = event-data() -> ("NewVal"=w342:bool)  [unwired: 1 in, 5 out]
        n312 = case shown="真" w342 {
          frame False {
          }
          frame True {
            n313 = local write "单体电压"(3.3 ("单体电压")) -> ()
            n314 = local write "电压个数"(60.0 ("电压个数")) -> ()
            n315 = local write "从板总电压"(200.0 ("总电压")) -> ()
            n316 = local write "位置"(10 ("位置")) -> ()
            n317 = local write "总电流"(200.0 ("总电流")) -> ()
            n318 = local write "外总压"(300.0 ("外总压")) -> ()
            n319 = local write "位置"(5 ("位置")) -> ()
            n320 = local write "平均电流"(150.0 ("平均电流")) -> ()
            n321 = local write "最大电压"(3.4 ("最大电压")) -> ()
            n322 = local write "最小电压"(3.36 ("最小电压")) -> ()
            n323 = local write "板号               单体电压          电压个数"(dbl[][] [[1.0, 3.3, 60.0], [2.0, 3.3, 60.0], [3.0, 3.3, 60.0], [4.0, 3.3, 60.0], [5.0, 3.3, 60.0], [6.0, 3.3, 60.0], [7.0, 3.3, 60.0], [8.0, 3.3, 60.0], [10.0, 3.3, 60.0], [11.0, 3.3, 60.0], [12.0, 3.3, 60.0], [13.0, 3.3, 60.0], [14.0, 3.3, 60.0], [15.0, 3.3, 60.0], [16.0, 3.3, 60.0], [17.0, 3.3, 60.0], [18.0, 3.3, 60.0], [19.0, 3.3, 60.0], [20.0, 3.3, 60.0]] ("单体电压          电压个数")) -> ()
            n324 = local write "温度个数"(10.0 ("温度个数")) -> ()
            n325 = local write "位置"(8 ("位置")) -> ()
            n326 = local write "位置"(4 ("位置")) -> ()
            n327 = local write "最大温度"(27.0 ("最大温度")) -> ()
            n328 = local write "最小温度"(25.0 ("最小温度")) -> ()
            n329 = local write "温度"(25.0 ("温度")) -> ()
            n330 = local write "硬件故障"("0000000000000000" ("硬件故障")) -> ()
            n331 = local write "板号          温度              温度个数"(dbl[][] [[1.0, 25.0, 10.0], [2.0, 25.0, 10.0], [3.0, 25.0, 10.0], [4.0, 25.0, 10.0], [5.0, 25.0, 10.0], [6.0, 25.0, 10.0], [7.0, 25.0, 10.0], [8.0, 25.0, 10.0], [10.0, 25.0, 10.0], [11.0, 25.0, 10.0], [12.0, 25.0, 10.0], [13.0, 25.0, 10.0], [14.0, 25.0, 10.0], [15.0, 25.0, 10.0], [16.0, 25.0, 10.0], [17.0, 25.0, 10.0], [18.0, 25.0, 10.0], [19.0, 25.0, 10.0], [20.0, 25.0, 10.0]] ("单体电压          电压个数")) -> ()
            n332 = local write "充电总安时"(0.0 ("充电总安时")) -> ()
            n333 = local write "放电总安时"(0.0 ("放电总安时")) -> ()
            n334 = local write "总电压 2"(300.0 ("总电压 2")) -> ()
            n335 = local write "总电流 2"(200.0 ("总电流 2")) -> ()
            n336 = local write "外总压 2"(300.0 ("外总压 2")) -> ()
            n337 = local write "平均电流 2"(150.0 ("平均电流 2")) -> ()
          }
        }
      }
      event "单体电压": Value Change {
        n338 = event-data() -> ()  [unwired: 1 in, 6 out]
        n339 = local read "板号               单体电压          电压个数"() -> (w373:dbl[][])
        n340 = local read "单体电压"() -> (w371:dbl)
        n341 = for {
          N: 20 -> [_]
          tunnel: w371 -> [w374]
          tunnel: [w374] -> w369 mode=indexing
        }
        n342 = Replace Array Subset(array=w373, new element=w369, index (col)=1 ("禁用的索引 (列)")) -> (w368:dbl[][])  [unwired: 1 in]
        n343 = local write "板号               单体电压          电压个数"(w368) -> ()
      }
      event "温度": Value Change {
        n344 = event-data() -> ()  [unwired: 1 in, 6 out]
        n345 = local read "板号          温度              温度个数"() -> (w377:dbl[][])
        n346 = local read "温度"() -> (w375:dbl)
        n347 = for {
          N: 20 -> [_]
          tunnel: w375 -> [w381]
          tunnel: [w381] -> w378 mode=indexing
        }
        n348 = Replace Array Subset(array=w377, new element=w378, index (col)=1 ("禁用的索引 (列)")) -> (w376:dbl[][])  [unwired: 1 in]
        n349 = local write "板号          温度              温度个数"(w376) -> ()
      }
      event "温度个数": Value Change {
        n350 = event-data() -> ()  [unwired: 1 in, 6 out]
        n351 = local read "温度个数"() -> (w382:dbl)
        n352 = local read "板号          温度              温度个数"() -> (w384:dbl[][])
        n353 = for {
          N: 20 -> [_]
          tunnel: w382 -> [w388]
          tunnel: [w388] -> w385 mode=indexing
        }
        n354 = Replace Array Subset(array=w384, new element=w385, index (col)=2 ("禁用的索引 (列)")) -> (w383:dbl[][])  [unwired: 1 in]
        n355 = local write "板号          温度              温度个数"(w383) -> ()
      }
      event "电压个数": Value Change {
        n356 = event-data() -> ()  [unwired: 1 in, 6 out]
        n357 = local read "板号               单体电压          电压个数"() -> (w394:dbl[][])
        n358 = local read "电压个数"() -> (w389:dbl)
        n359 = for {
          N: 20 -> [_]
          tunnel: w389 -> [w395]
          tunnel: [w395] -> w391 mode=indexing
        }
        n360 = Replace Array Subset(array=w394, new element=w391, index (col)=2 ("禁用的索引 (列)")) -> (w390:dbl[][])  [unwired: 1 in]
        n361 = local write "板号               单体电压          电压个数"(w390) -> ()
      }
      event "停止": Value Change {
        n362 = event-data() -> ("NewVal"=w396:bool)  [unwired: 1 in, 5 out]
        "Stop" <- w396
      }
      event Panel Close {
        n363 = event-data() -> ()  [unwired: 1 in, 4 out]
        n364 = local write "Stop"(TRUE ("Stop")) -> ()
      }
      event "内部CAN发送通道": Value Change {
        n365 = event-data() -> ("NewVal"=w399:u16)  [unwired: 1 in, 5 out]
        n366 = case shown="1" w399 {
          frame 0, Default {
          }
          frame 1 {
            n367 = global read "EV05全局变量1.vi" "设备索引号"() -> (w401:u16)
            n368 = global read "EV05全局变量1.vi" "波特率"() -> (w400:u16)
            n369 = global read "EV05全局变量1.vi" "CAN卡类型"() -> (w402:u32)
            n370 = local read "内部CAN发送通道"() -> (w403:u16)
            n371 = call "CAN_Init-donotOpen.vi"("设备类型"=w402, "设备索引"=w401, "波特率"=w400, "CAN路数"=w403) -> ()  [unwired: 14 in, 2 out]
          }
        }
      }
      event "自定信息CAN发送通道": Value Change {
        n372 = event-data() -> ("NewVal"=w404:u16)  [unwired: 1 in, 5 out]
        n373 = case shown="1" w404 {
          frame 0, Default {
          }
          frame 1 {
            n374 = local read "自定信息CAN发送通道"() -> (w406:u16)
            n375 = global read "EV05全局变量1.vi" "设备索引号"() -> (w407:u16)
            n376 = global read "EV05全局变量1.vi" "CAN卡类型"() -> (w408:u32)
            n377 = call "CAN_Init-donotOpen.vi"("设备类型"=w408, "设备索引"=w407, "波特率"="自定义信息CAN波特率", "CAN路数"=w406) -> ()  [unwired: 14 in, 2 out]
          }
        }
      }
      event "自定义信息CAN波特率": Value Change {
        n378 = event-data() -> ("NewVal"=w409:enum16{"250Kbps", "500Kbps"})  [unwired: 1 in, 5 out]
        n379 = local read "自定信息CAN发送通道"() -> (w410:u16)
        n380 = global read "EV05全局变量1.vi" "设备索引号"() -> (w411:u16)
        n381 = global read "EV05全局变量1.vi" "CAN卡类型"() -> (w412:u32)
        n382 = call "CAN_Init-donotOpen.vi"("设备类型"=w412, "设备索引"=w411, "波特率"=w409, "CAN路数"=w410) -> ()  [unwired: 14 in, 2 out]
      }
    }
  }
  n383 = while {
    stop <- w413 stop-if-true
    n384 = Wait (ms)(milliseconds to wait=u32 50 ("等待时间（毫秒）")) -> ()  [unwired: 1 out]
    n385 = case shown="真" TRUE {
      frame False {
      }
      frame True {
        n386 = local read "从板个数"() -> (w416:T1)
        n387 = Increment(x=w416) -> (x+1=w417:T1)
        n388 = for {
          N: w417 -> [_]
          i -> [w418]
          n389 = stacked-sequence {
            tunnel: w418 -> [w419 _ w668 w728]
            frame #0 {
              n390 = for {
                N: 6 -> [_]
                tunnel: w419 -> [w421]
                i -> [w430]
                n391 = case shown="3" w430 {
                  tunnel: [w436 w478 w516 w525 w547 w602] -> w425
                  tunnel: [w450 w453 w488 w523 w597 w599] -> w426
                  tunnel: w421 -> [w431 w452 w483 w517 w526 w600]
                  frame 0, Default {
                    n392 = call "输入分辨率计算-EV05.vi"("1字节?"=FALSE, "数值 2"="外总压", "数值"="从板总电压", "分辨率"=0.1) -> ("低字节 2"=w439:dbl, "高字节 2"=w440:dbl, "低字节"=w443:dbl, "高字节1"=w444:dbl)  [unwired: 4 in]
                    n393 = call "输入分辨率计算-EV05.vi"("1字节?"=FALSE, "数值 2"="平均电流", "数值"="总电流", "偏移量"=-3000.0, "分辨率"=0.1) -> ("低字节 2"=w437:dbl, "高字节 2"=w438:dbl, "低字节"=w441:dbl, "高字节1"=w442:dbl)  [unwired: 3 in]
                    n394 = Build Array(w444, w443, w442, w441, w440, w439, w438, w437) -> (w436:dbl[])
                    n395 = Add(x=67211521, y=w431) -> (x+y=w450:i32)
                  }
                  frame 1 {
                    n396 = Quotient & Remainder(x="位置", y=256) -> (x-y*floor(x/y)=w470:i32, floor(x/y)=w473:i32)
                    n397 = Quotient & Remainder(x="位置", y=256) -> (x-y*floor(x/y)=w455:i32, floor(x/y)=w461:i32)
                    n398 = call "输入分辨率计算-EV05.vi"("1字节?"=FALSE, "数值 2"="最小电压", "数值"="最大电压", "分辨率"=0.001) -> ("低字节 2"=w462:dbl, "高字节 2"=w463:dbl, "低字节"=w464:dbl, "高字节1"=w465:dbl)  [unwired: 4 in]
                    n399 = call "二进制解析-8.6.vi"("索引"=4, "数值"=w470) -> ("低位子数组"=w458:i32[], "高位子数组"=w468:i32[])  [unwired: 1 in, 1 out]
                    n400 = call "二进制解析-8.6.vi"("索引"=4, "数值"=w473) -> ("低位子数组"=w469:i32[])  [unwired: 1 in, 2 out]
                    n401 = call "二进制解析-8.6.vi"("索引"=4, "数值"=w461) -> ("低位子数组"=w459:i32[])  [unwired: 1 in, 2 out]
                    n402 = Insert Into Array(array=w458, new element=w459) -> (w457:i32[])  [unwired: 1 in]
                    n403 = Insert Into Array(array=w469, new element=w468) -> (w467:i32[])  [unwired: 1 in]
                    n404 = call "数值二进制转十进制-8.6.vi"("子数组"=w457) -> ("十进制数值"=w456:i32)  [unwired: 4 in]
                    n405 = call "数值二进制转十进制-8.6.vi"("子数组"=w467) -> ("十进制数值"=w466:i32)  [unwired: 4 in]
                    n406 = Add(x=67277057, y=w452) -> (x+y=w453:i32)
                    n407 = Build Array(w465, w464, w463, w462, w466, w456, w455) -> (w478:dbl[])
                  }
                  frame 2 {
                    n408 = local read "板号          温度              温度个数"() -> (w485:dbl[][])
                    n409 = Index Array(array=w485, index (col)=2 ("禁用的索引 (列)")) -> (element=w486:dbl[])  [unwired: 1 in]
                    n410 = Index Array(array=w486, index=w483) -> (element=w484:dbl)
                    n411 = Quotient & Remainder(x="位置", y=256) -> (x-y*floor(x/y)=w505:i32, floor(x/y)=w508:i32)
                    n412 = Quotient & Remainder(x="位置", y=256) -> (x-y*floor(x/y)=w490:i32, floor(x/y)=w501:i32)
                    n413 = call "二进制解析-8.6.vi"("索引"=4, "数值"=w505) -> ("低位子数组"=w498:i32[], "高位子数组"=w503:i32[])  [unwired: 1 in, 1 out]
                    n414 = call "二进制解析-8.6.vi"("索引"=4, "数值"=w508) -> ("低位子数组"=w504:i32[])  [unwired: 1 in, 2 out]
                    n415 = call "二进制解析-8.6.vi"("索引"=4, "数值"=w501) -> ("低位子数组"=w499:i32[])  [unwired: 1 in, 2 out]
                    n416 = Insert Into Array(array=w498, new element=w499) -> (w497:i32[])  [unwired: 1 in]
                    n417 = Insert Into Array(array=w504, new element=w503) -> (w502:i32[])  [unwired: 1 in]
                    n418 = call "输入分辨率计算-EV05.vi"("1字节?"=TRUE, "数值 2"="最小温度", "数值"="最大温度", "偏移量"=-40.0, "分辨率"=1.0) -> ("高字节 2"=w509:dbl, "高字节1"=w510:dbl)  [unwired: 3 in, 2 out]
                    n419 = call "数值二进制转十进制-8.6.vi"("子数组"=w497) -> ("十进制数值"=w491:i32)  [unwired: 4 in]
                    n420 = call "数值二进制转十进制-8.6.vi"("子数组"=w502) -> ("十进制数值"=w492:i32)  [unwired: 4 in]
                    n421 = Add(x=67342593, y=w483) -> (x+y=w488:i32)
                    n422 = Build Array(w510, w509, w492, w491, w490, w484) -> (w516:dbl[])
                  }
                  frame 5 {
                    w518 = 0.0 ("元素")
                    n423 = local read "板号               单体电压          电压个数"() -> (w520:dbl[][])
                    n424 = Index Array(array=w520, index (col)=2 ("禁用的索引 (列)")) -> (element=w521:dbl[])  [unwired: 1 in]
                    n425 = Index Array(array=w521, index=w517) -> (element=w519:dbl)
                    n426 = Add(x=67408129, y=w517) -> (x+y=w523:i32)
                    n427 = Build Array(w518, w518, w518, w518, w518, w518, w518, w519) -> (w525:dbl[])
                  }
                  frame 3 {
                    w529 = "00" ("字符串")
                    w546 = 0 ("元素")
                    w576 = 2
                    n428 = local read "CPU内部FLASH存储器故障"() -> (w586:enum16{"无", "一级", "二级", "三级"})
                    n429 = local read "系统外扩时钟模块故障"() -> (w590:enum16{"无", "一级", "二级", "三级"})
                    n430 = local read "内总压检测模块故障"() -> (w592:enum16{"无", "一级", "二级", "三级"})
                    n431 = local read "外总压检测模块故障"() -> (w591:enum16{"无", "一级", "二级", "三级"})
                    n432 = local read "45db041存储器故障"() -> (w587:enum16{"无", "一级", "二级", "三级"})
                    n433 = local read "CAN4通讯模块故障"() -> (w584:enum16{"无", "一级", "二级", "三级"})
                    n434 = local read "CAN0通讯模块故障"() -> (w583:enum16{"无", "一级", "二级", "三级"})
                    n435 = local read "CAN1通讯模块故障"() -> (w582:enum16{"无", "一级", "二级", "三级"})
                    n436 = local read "电压检测模块故障"() -> (w596:enum16{"无", "一级", "二级", "三级"})
                    n437 = local read "温度检测模块故障"() -> (w595:enum16{"无", "一级", "二级", "三级"})
                    n438 = local read "电流检测模块故障"() -> (w594:enum16{"无", "一级", "二级", "三级"})
                    n439 = local read "绝缘检测模块故障"() -> (w593:enum16{"无", "一级", "二级", "三级"})
                    n440 = local read "充电均衡模块故障"() -> (w581:enum16{"无", "一级", "二级", "三级"})
                    n441 = local read "放电均衡模块故障"() -> (w580:enum16{"无", "一级", "二级", "三级"})
                    n442 = local read "CPU内部EE故障"() -> (w589:enum16{"无", "一级", "二级", "三级"})
                    n443 = local read "EE存储器故障"() -> (w588:enum16{"无", "一级", "二级", "三级"})
                    n444 = local read "DO模块故障"() -> (w577:enum16{"无", "一级", "二级", "三级"})
                    n445 = local read "DI模块故障"() -> (w578:enum16{"无", "一级", "二级", "三级"})
                    n446 = local read "软件故障"() -> (w579:enum16{"无", "一级", "二级", "三级"})
                    n447 = local read "CPU故障"() -> (w585:enum16{"无", "一级", "二级", "三级"})
                    n448 = call "二进制解析-8.6.vi"("索引"=w576, "数值"=w586) -> ("低位子数组"=w559:i32[])  [unwired: 1 in, 2 out]
                    n449 = call "二进制解析-8.6.vi"("索引"=w576, "数值"=w582) -> ("低位子数组"=w555:i32[])  [unwired: 1 in, 2 out]
                    n450 = call "二进制解析-8.6.vi"("索引"=w576, "数值"=w580) -> ("低位子数组"=w550:i32[])  [unwired: 1 in, 2 out]
                    n451 = call "二进制解析-8.6.vi"("索引"=w576, "数值"=w579) -> ("低位子数组"=w551:i32[])  [unwired: 1 in, 2 out]
                    n452 = call "二进制解析-8.6.vi"("索引"=w576, "数值"=w578) -> ("低位子数组"=w543:i32[])  [unwired: 1 in, 2 out]
                    n453 = call "二进制解析-8.6.vi"("索引"=w576, "数值"=w577) -> ("低位子数组"=w544:i32[])  [unwired: 1 in, 2 out]
                    n454 = call "二进制解析-8.6.vi"("索引"=w576, "数值"=w594) -> ("低位子数组"=w568:i32[])  [unwired: 1 in, 2 out]
                    n455 = call "二进制解析-8.6.vi"("索引"=w576, "数值"=w588) -> ("低位子数组"=w557:i32[])  [unwired: 1 in, 2 out]
                    n456 = call "二进制解析-8.6.vi"("索引"=w576, "数值"=w587) -> ("低位子数组"=w558:i32[])  [unwired: 1 in, 2 out]
                    n457 = call "二进制解析-8.6.vi"("索引"=w576, "数值"=w585) -> ("低位子数组"=w560:i32[])  [unwired: 1 in, 2 out]
                    n458 = call "二进制解析-8.6.vi"("索引"=w576, "数值"=w584) -> ("低位子数组"=w553:i32[])  [unwired: 1 in, 2 out]
                    n459 = call "二进制解析-8.6.vi"("索引"=w576, "数值"=w583) -> ("低位子数组"=w554:i32[])  [unwired: 1 in, 2 out]
                    n460 = call "二进制解析-8.6.vi"("索引"=w576, "数值"=w581) -> ("低位子数组"=w549:i32[])  [unwired: 1 in, 2 out]
                    n461 = call "二进制解析-8.6.vi"("索引"=w576, "数值"=w596) -> ("低位子数组"=w566:i32[])  [unwired: 1 in, 2 out]
                    n462 = call "二进制解析-8.6.vi"("索引"=w576, "数值"=w595) -> ("低位子数组"=w567:i32[])  [unwired: 1 in, 2 out]
                    n463 = call "二进制解析-8.6.vi"("索引"=w576, "数值"=w593) -> ("低位子数组"=w569:i32[])  [unwired: 1 in, 2 out]
                    n464 = call "二进制解析-8.6.vi"("索引"=w576, "数值"=w590) -> ("低位子数组"=w564:i32[])  [unwired: 1 in, 2 out]
                    n465 = call "二进制解析-8.6.vi"("索引"=w576, "数值"=w592) -> ("低位子数组"=w562:i32[])  [unwired: 1 in, 2 out]
                    n466 = call "二进制解析-8.6.vi"("索引"=w576, "数值"=w591) -> ("低位子数组"=w563:i32[])  [unwired: 1 in, 2 out]
                    n467 = call "二进制解析-8.6.vi"("索引"=w576, "数值"=w589) -> ("低位子数组"=w565:i32[])  [unwired: 1 in, 2 out]
                    n468 = Insert Into Array(array=w565, new element #1=w564, new element #2=w563, new element #3=w562) -> (w570:i32[])  [unwired: 1 in]
                    n469 = Insert Into Array(array=w569, new element #1=w568, new element #2=w567, new element #3=w566) -> (w575:i32[])  [unwired: 1 in]
                    n470 = Insert Into Array(array=w560, new element #1=w559, new element #2=w558, new element #3=w557) -> (w561:i32[])  [unwired: 1 in]
                    n471 = Insert Into Array(array=w555, new element #1=w554, new element #2=w553) -> (w556:i32[])  [unwired: 1 in]
                    n472 = Insert Into Array(array=w551, new element #1=i32[] [0, 0], new element #2=w550, new element #3=w549) -> (w552:i32[])  [unwired: 1 in]
                    n473 = Insert Into Array(array=w544, new element=w543) -> (w545:i32[])  [unwired: 1 in]
                    n474 = call "数值二进制转十进制-8.6.vi"("子数组"=w570) -> ("十进制数值"=w537:i32)  [unwired: 4 in]
                    n475 = call "数值二进制转十进制-8.6.vi"("子数组"=w575) -> ("十进制数值"=w571:i32)  [unwired: 4 in]
                    n476 = call "数值二进制转十进制-8.6.vi"("子数组"=w561) -> ("十进制数值"=w536:i32)  [unwired: 4 in]
                    n477 = call "数值二进制转十进制-8.6.vi"("子数组"=w556) -> ("十进制数值"=w535:i32)  [unwired: 4 in]
                    n478 = call "数值二进制转十进制-8.6.vi"("子数组"=w552) -> ("十进制数值"=w534:i32)  [unwired: 4 in]
                    n479 = call "数值二进制转十进制-8.6.vi"("子数组"=w545) -> ("十进制数值"=w533:i32)  [unwired: 4 in]
                    n480 = Number To Hexadecimal String(1:i16 2 ("宽度(-)"), 2:w537) -> (0:w532:string)
                    n481 = Number To Hexadecimal String(1:i16 2 ("宽度(-)"), 2:w571) -> (0:w573:string)
                    n482 = Number To Hexadecimal String(1:i16 2 ("宽度(-)"), 2:w535) -> (0:w530:string)
                    n483 = Number To Hexadecimal String(1:i16 2 ("宽度(-)"), 2:w536) -> (0:w531:string)
                    n484 = Number To Hexadecimal String(1:i16 2 ("宽度(-)"), 2:w534) -> (0:w528:string)
                    n485 = Number To Hexadecimal String(1:i16 2 ("宽度(-)"), 2:w533) -> (0:w527:string)
                    n486 = Build Array(w571, w537, w536, w535, w546, w534, w546, w533) -> (w547:i32[])
                    n487 = Concatenate Strings(w573, w532, w531, w530, w529, w528, w529, w527) -> (→"硬件故障":string)
                    n488 = Add(x=67997953, y=w526) -> (x+y=w597:i32)
                  }
                  frame 4 {
                    w603 = 0
                    n489 = local read "LIFE"() -> (w604:i32)
                    n490 = Build Array(w603, w603, w603, w603, w603, w603, w603, w604) -> (w602:i32[])
                    n491 = Increment(x=w604) -> (x+1=w609:i32)
                    n492 = Greater Or Equal?(x=w609, y=255) -> (x >= y?=w606:bool)
                    n493 = Select(t=1 ("y"), s=w606, f=w609) -> (s? t:f=w608:i32)
                    n494 = local write "LIFE"(w608) -> ()
                    n495 = Add(x=83836673, y=w600) -> (x+y=w599:i32)
                  }
                }
                n496 = local read "内部CAN发送通道"() -> (w422:u16)
                n497 = global read "EV05全局变量1.vi" "设备索引号"() -> (w428:u16)
                n498 = global read "EV05全局变量1.vi" "CAN卡类型"() -> (w427:u32)
                n499 = Wait Until Next ms Multiple(millisecond multiple=u32 10 ("毫秒倍数")) -> ()  [unwired: 1 out]
                n500 = call "transmit-8.6.vi"("can卡类型"=w427, "设备索引号"=w428, "CAN端口"=w422, "ID"=w426, "SendType"=u8 2, "Data"=w425) -> ("发送成功"=→"发送成功":bool)  [unwired: 3 in, 10 out]
              }
            }
            frame #1 {
              n501 = local read "发送?"() -> (w610:bool)
              n502 = case shown="真" w610 {
                frame False {
                }
                frame True {
                  n503 = for {
                    N: 2 -> [_]
                    i -> [w618]
                    n504 = case shown="0, 默认" w618 {
                      tunnel: [w620 w655] -> w614
                      tunnel: [67146046 67473726] -> w613
                      frame 0, Default {
                        n505 = local read "平均电流 2"() -> (w624:dbl)
                        n506 = local read "总电压 2"() -> (w621:dbl)
                        n507 = local read "外总压 2"() -> (w622:dbl)
                        n508 = local read "总电流 2"() -> (w623:dbl)
                        n509 = call "输入分辨率计算-EV05.vi"("1字节?"=FALSE, "数值 2"=w622, "数值"=w621, "分辨率"=0.1) -> ("低字节 2"=w635:dbl, "高字节 2"=w634:dbl, "低字节"=w631:dbl, "高字节1"=w630:dbl)  [unwired: 4 in]
                        n510 = call "输入分辨率计算-EV05.vi"("1字节?"=FALSE, "数值 2"=w624, "数值"=w623, "偏移量"=-3000.0, "分辨率"=0.1) -> ("低字节 2"=w637:dbl, "高字节 2"=w636:dbl, "低字节"=w633:dbl, "高字节1"=w632:dbl)  [unwired: 3 in]
                        n511 = Build Array(w630, w631, w632, w633, w634, w635, w636, w637) -> (w620:dbl[])
                      }
                      frame 1 {
                        n512 = local read "放电总安时"() -> (w658:dbl)
                        n513 = local read "充电总安时"() -> (w659:dbl)
                        n514 = call "输入分辨率计算-EV05.vi"("1字节?"=FALSE, "数值 2"=w658, "数值"=w659, "分辨率"=0.1) -> ("低字节 2"=w641:dbl, "高字节 2"=w642:dbl, "低字节"=w649:dbl, "高字节1"=w652:dbl)  [unwired: 4 in]
                        n515 = Quotient & Remainder(x=w642, y=256.0) -> (x-y*floor(x/y)=w640:dbl, floor(x/y)=w645:dbl)
                        n516 = Quotient & Remainder(x=w652, y=256.0) -> (x-y*floor(x/y)=w648:dbl, floor(x/y)=w650:dbl)
                        n517 = Quotient & Remainder(x=w645, y=256.0) -> (x-y*floor(x/y)=w638:dbl, floor(x/y)=w639:dbl)
                        n518 = Quotient & Remainder(x=w650, y=256.0) -> (x-y*floor(x/y)=w647:dbl, floor(x/y)=w646:dbl)
                        n519 = Build Array(w646, w647, w648, w649, w639, w638, w640, w641) -> (w655:dbl[])
                      }
                    }
                    n520 = local read "内部CAN发送通道"() -> (w612:u16)
                    n521 = global read "EV05全局变量1.vi" "CAN卡类型"() -> (w617:u32)
                    n522 = global read "EV05全局变量1.vi" "设备索引号"() -> (w616:u16)
                    n523 = call "transmit-8.6.vi"("can卡类型"=w617, "设备索引号"=w616, "CAN端口"=w612, "ID"=w613, "SendType"=u8 2, "Data"=w614) -> ()  [unwired: 3 in, 11 out]
                  }
                }
              }
            }
            frame #2 {
              # "0x80091xx"
              n524 = local read "板号               单体电压          电压个数"() -> (w671:dbl[][])
              n525 = Index Array(array=w671, index (col)=1 ("禁用的索引 (列)")) -> (element=w669:dbl[])  [unwired: 1 in]
              n526 = Index Array(array=w671, index (col)=2 ("禁用的索引 (列)")) -> (element=w676:dbl[])  [unwired: 1 in]
              n527 = Index Array(array=w669, index=w668) -> (element=w667:dbl)
              n528 = Index Array(array=w676, index=w668) -> (element=w672:dbl)
              n529 = Quotient & Remainder(x=w672, y=4.0) -> (x-y*floor(x/y)=w674:dbl, floor(x/y)=w673:dbl)
              n530 = Multiply(x=w667, y=1000.0) -> (x*y=w665:dbl)
              n531 = local read "发送单体电压递增1mv"() -> (w660:bool)
              n532 = case shown="1, 默认" w674 {
                tunnel: w673 -> [w679 w680]
                tunnel: [w678 w680] -> w661
                frame 1, Default {
                  n533 = Increment(x=w679) -> (x+1=w678:dbl)
                }
                frame 0 {
                }
              }
              n534 = To Unsigned Word Integer(number=w665) -> (unsigned 16bit integer=w664:u16)
              n535 = Add(x=w664, y=u16 32768) -> (x+y=w662:u16)
              n536 = for {
                N: w661 -> [_]
                tunnel: w668 -> [w703]
                tunnel: w662 -> [w688]
                tunnel: w660 -> [w690]
                i -> [w682]
                n537 = To Unsigned Word Integer(number=w682) -> (unsigned 16bit integer=w681:u16)
                n538 = Multiply(x=u16 4, y=w681) -> (x*y=w683:u16)
                n539 = case shown="真" w690 {
                  tunnel: w688 -> [w710 w713]
                  tunnel: w683 -> [_ w720]
                  tunnel: [w710 w719] -> w687
                  tunnel: [w710 w718] -> w686
                  tunnel: [w710 w712] -> w685
                  tunnel: [w710 w711] -> w684
                  frame False {
                  }
                  frame True {
                    n540 = Increment(x=w720) -> (x+1=w717:u16)
                    n541 = Increment(x=w717) -> (x+1=w716:u16)
                    n542 = Increment(x=w716) -> (x+1=w715:u16)
                    n543 = Increment(x=w715) -> (x+1=w714:u16)
                    n544 = Add(x=w716, y=w713) -> (x+y=w718:u16)
                    n545 = Add(x=w717, y=w713) -> (x+y=w719:u16)
                    n546 = Add(x=w715, y=w713) -> (x+y=w712:u16)
                    n547 = Add(x=w713, y=w714) -> (x+y=w711:u16)
                  }
                }
                n548 = Split Number(x=w687) -> (hi(x)=w700:u8, lo(x)=w699:u8)
                n549 = Split Number(x=w686) -> (hi(x)=w698:u8, lo(x)=w697:u8)
                n550 = Split Number(x=w685) -> (hi(x)=w696:u8, lo(x)=w695:u8)
                n551 = Split Number(x=w684) -> (hi(x)=w694:u8, lo(x)=w693:u8)
                n552 = Multiply(x=w681, y=65536) -> (x*y=w701:i32)
                n553 = Build Array(w700, w699, w698, w697, w696, w695, w694, w693) -> (w692:u8[])
                n554 = local read "内部CAN发送通道"() -> (w709:u16)
                n555 = Compound Arithmetic op=ADD(w701, 134254849, w703) -> (w704:i32)
                n556 = global read "EV05全局变量1.vi" "CAN卡类型"() -> (w708:u32)
                n557 = global read "EV05全局变量1.vi" "设备索引号"() -> (w707:u16)
                n558 = call "transmit-8.6.vi"("can卡类型"=w708, "设备索引号"=w707, "CAN端口"=w709, "ID"=w704, "SendType"=u8 2, "Data"=w692) -> ()  [unwired: 3 in, 11 out]
                n559 = Wait (ms)(milliseconds to wait=u32 5 ("等待时间（毫秒）")) -> ()  [unwired: 1 out]
              }
            }
            frame #3 {
              # "0x80091xx"
              n560 = local read "板号          温度              温度个数"() -> (w726:dbl[][])
              n561 = Index Array(array=w726, index (col)=1 ("禁用的索引 (列)")) -> (element=w729:dbl[])  [unwired: 1 in]
              n562 = Index Array(array=w726, index (col)=2 ("禁用的索引 (列)")) -> (element=w735:dbl[])  [unwired: 1 in]
              n563 = Index Array(array=w729, index=w728) -> (element=w725:dbl)
              n564 = Index Array(array=w735, index=w728) -> (element=w731:dbl)
              n565 = Quotient & Remainder(x=w731, y=4.0) -> (x-y*floor(x/y)=w733:dbl, floor(x/y)=w732:dbl)
              n566 = Add(x=w725, y=40.0) -> (x+y=w723:dbl)
              n567 = case shown="1, 默认" w733 {
                tunnel: w732 -> [w738 w739]
                tunnel: [w737 w739] -> w727
                frame 1, Default {
                  n568 = Increment(x=w738) -> (x+1=w737:dbl)
                }
                frame 0 {
                }
              }
              n569 = To Unsigned Byte Integer(number=w723) -> (unsigned 8bit integer=w722:u8)
              n570 = local read "发送温度递增1度"() -> (w721:bool)
              n571 = for {
                N: w727 -> [_]
                tunnel: w728 -> [w748]
                tunnel: w722 -> [w743]
                tunnel: w721 -> [w742]
                i -> [w741]
                n572 = To Unsigned Byte Integer(number=w741) -> (unsigned 8bit integer=w740:u8)
                n573 = case shown="真" w742 {
                  tunnel: [w755 w766] -> w745
                  tunnel: w743 -> [w758 w765]
                  tunnel: w740 -> [w760 _]
                  frame True {
                    n574 = Multiply(x=w760, y=u8 8) -> (x*y=w756:u8)
                    n575 = for {
                      N: 8 -> [_]
                      tunnel: w758 -> [w764]
                      tunnel: w756 -> [w763]
                      tunnel: [w761] -> w755 mode=indexing
                      i -> [w762]
                      n576 = Compound Arithmetic op=ADD(w764, w763, w762) -> (w761:i32)
                    }
                  }
                  frame False {
                    n577 = Build Array(w765, w765, w765, w765, w765, w765, w765, w765) -> (w766:u8[])
                  }
                }
                n578 = Multiply(x=w740, y=65536) -> (x*y=w746:i32)
                n579 = Compound Arithmetic op=ADD(w746, 268472577, w748) -> (w749:i32)
                n580 = local read "内部CAN发送通道"() -> (w754:u16)
                n581 = global read "EV05全局变量1.vi" "CAN卡类型"() -> (w753:u32)
                n582 = global read "EV05全局变量1.vi" "设备索引号"() -> (w752:u16)
                n583 = call "transmit-8.6.vi"("can卡类型"=w753, "设备索引号"=w752, "CAN端口"=w754, "ID"=w749, "SendType"=u8 2, "Data"=w745) -> ()  [unwired: 3 in, 11 out]
                n584 = Wait (ms)(milliseconds to wait=u32 5 ("等待时间（毫秒）")) -> ()  [unwired: 1 out]
              }
            }
          }
        }
      }
    }
    n585 = local read "Stop"() -> (w413:bool)
  }
  n586 = local write "内部CAN发送通道"(w1) -> ()
